vi "Periodic Tasks.vi"(8 "error in":errorcluster) -> ()   [LabVIEW 2011]
doc: "This VI runs in parallel to other tasks. It can contain as many user-defined periodic loops as you need. These can carry out PID or other sorts of timed response."
uses:
  <vilib>/Rock Robotics/SystemInterfaces/Typedef/FPGA_TypedefDigitalModule.ctl
  ADXL345 I2C Range.ctl
  <vilib>/Rock Robotics/SystemInterfaces/Utilities/FPGA_UtilitiesLED Source.ctl
  <vilib>/Rock Robotics/SystemInterfaces/Utilities/FPGA_UtilitiesLED State.ctl
  <vilib>/Rock Robotics/WPI/Relay/WPI_RelayValue.ctl
  Robot Global Data.vi
  <vilib>/Utility/file.llb/Read From Spreadsheet File (string).vi
  <vilib>/addons/control/pid/pid.llb/PID (DBL).vi
  <vilib>/Rock Robotics/WPI/RobotDrive/WPI_RobotDriveArcadeDrive_Standard(NoSaturation).vi
  <vilib>/addons/control/pid/pid.llb/PID Output Rate Limiter (DBL).vi
  ADXL345 I2C Axis.ctl
  <vilib>/addons/control/pid/NI_PID_pid.lvlib
  <vilib>/Utility/file.llb/Write To Spreadsheet File (DBL).vi
panel:
  in  "BB A Delay":dbl=0.15
  in  "Coll Loop TIme":u32=50
  in  "Save Data":bool
  in  "Tip Tol 2":dbl
  in  "K Deriv 2":dbl
  in  "K Prop 2":dbl
  in  "Reset Sonar 4":bool
  in  "Reset Sonar 3":bool
  in  "Motor C":dbl=-1.0
  in  "time":dbl
  in  "Dial":i64(knob)=50 scale=0.0..500.0
  in  "error":dbl(knob) scale=-0.5..0.5
  out "L Sonar":cluster{dbl, "Filtered":dbl}(graph)
  out "R Sonar":cluster{dbl, "Filtered":dbl}(graph)
  out "Gain (VoltsPerDegree/Second)":dbl
  out "Gain":dbl
  out "Left Enc":dbl
  out "Right Enc":dbl
  out "Right Wheel Encoder":dbl
  out "Left Wheel Encoder":dbl
  out "output 2":dbl format="%.2f"
  out "output":dbl format="%.2f"
  out "MAC Address":string
  out "Personality":string
  in  "Number Samples to Average":u8(knob)=30 min=1 max=128 scale=0.0..30.0
  in  "Minimum Rate":dbl(knob)=10.067348623787787 scale=0.0..20.0
  out "Angle":dbl
  in  "Tab Control":T1(tab)
  out "Z axis":dbl(slide) scale=-1.0..1.0
  out "Y AXIS":dbl(slide) scale=-1.0..1.0
  out "X AXIS":dbl(slide) scale=-1.0..1.0
  out "R Mode":bool
  out "L Mode":bool
  in  "Sonar Offset":dbl(knob)=-0.020166607778801193 scale=-20.0..20.0
  in  "Sonar Scale":dbl(knob)=102.7182978218157 scale=80.0..120.0
  in  "Rate Thresh":dbl(knob)=100.27914654140737 step=0.001 scale=0.0..200.0
  out "Right Sonar":dbl
  out "Left Sonar":dbl
  out "R Filtered":dbl
  out "L Filtered":dbl
  out "R OOR":bool
  out "L OOR":bool
  out "hi limit":dbl=70.0
  in  "Hyster":dbl=0.3 step=0.1
  out "Valid Target":bool
  out "Stable":bool
  out "Intake":bool
  out "Steering":bool
  in  "Close":dbl=13.0
  out "Close?":bool
  in  "DS time":dbl=2.0
  in  "x":dbl=12.0
  in  "Balance 2":dbl=0.07
  in  "Gain 2":dbl=0.6 step=0.05
  in  "Base":dbl=0.8 step=0.1
  out "Left Motor Sonar":dbl=36.0
  out "Right Motor Sonar":dbl=36.0
  in  "IR Delay (sec)":dbl(knob)=0.20745032848680972 scale=0.0..1.0
  in  "Intake Delay (sec)":dbl(knob)=0.15160369527651382 scale=0.0..1.0
  out "error":dbl
  out "dist":dbl
  out "Sonar State":i32
  in  "Reset Sonar":bool
  out "Kick State":i32
  in  "Sonar Loop":bool
  in  "ms multiple":u32=50
  in  "DIO Module":T2
  in  "Range":T3 items=["+/- 2 g", "+/- 4 g", "+/- 8 g", "+/- 16 g"]
  out "Z Axis Accel":dbl
  out "Y Axis Accel":dbl
  out "X Axis Accel":dbl
  in  "stop":bool
  out "Loop":i32
  out "X Axis":dbl(knob) scale=-2.0..2.0
  out "Y Axis":dbl(knob) scale=-2.0..2.0
  out "Z Axis":dbl(knob) scale=-2.0..2.0
  out "Up ?":bool
  out "K Prop":dbl=0.04035443158900818
  out "Balance":cluster{"setpoint":dbl, "GYRO":dbl}(graph)
  in  "Bal Tol":dbl=2.0
  in  "Coerce":dbl=0.5
  out "Drive":dbl
  out "In Tol?":bool
  out "Tip Tol":dbl=2.25 step=0.01
  in  "Motor Add":dbl=0.1
  out "Pitch Angle":dbl
  out "Gain (VoltsPerDegree/Second) 2":dbl
  in  "reset":bool=TRUE
  in  "DRIFT (Deg/sec)":dbl(knob) scale=-0.3..0.3
  out "K Deriv":dbl=0.001046187815623034
  out "K Prop 2":dbl
  out "K Deriv 2":dbl
  out "Motor Add":dbl
  out "Coerce":dbl
  out "Bal Tol":dbl
  out "Tip Tol 2":dbl
  in  "T Ang Mult":dbl=-44.91
  in  "Turret Home Position":dbl=-180.0
  out "Turret Home Adjust":dbl
  out "Turret Yaw":dbl
  out "Turret Home":bool
  out "Read Right Limit":dbl=30.0
  out "Read Left Limit":dbl=-185.0
  in  "Motor Cuttout":dbl=0.06
  out "Motor is Cut Out":bool
  out "Turret Enc":dbl
  in  "Set Left Comp":dbl=-190.0
  in  "Set Right Comp":dbl=30.0
  in  "Speed near Limit":dbl=0.2
  in  "Near Limit (deg)":dbl=10.0
  out "Motor Command":dbl=0.04
  out "Softstop Override":bool
  in  "Set Left Test":dbl=-205.0
  in  "Set Right Test":dbl=30.0
  out "Left Limit":bool
  out "Right Limit":bool
  out "PB":bool
  out "Left Output":dbl format="%.2f"
  out "Left PID Out":dbl(graph)
  out "Left Brake Control Response":cluster{"setpoint":dbl, "Angle":dbl}(graph)
  in  "Deriv 2":dbl(knob)=0.0006002534638116536 scale=0.0..0.01
  in  "Int 2":dbl(knob) scale=0.0..0.2
  in  "Prop 2":dbl(knob)=0.18717165980295236 scale=0.0..0.5
  out "Right Output":dbl format="%.2f"
  in  "Brake Motor Add":dbl=0.05
  in  "Brake Motor Deadband":dbl=0.1
  in  "Brake Bump":i64=1
  in  "Bump rate":dbl=400.0 format="%.2f"
  in  "Shooter Loop milliseconds":u32=20
  in  "Shooter Stable Tol (sec)":dbl(knob)=0.5029660632222493 scale=0.0..1.0
  out "Motor Command":dbl(slide) scale=0.0..1.0
  out "RPM In Tol ?":bool
  out "RPM Stable ?":bool
  out "Distance":dbl
  out "Frame":i32
  out "Angle 2":dbl
  out "Valid Target 2":bool
  in  "Momen Time (sec)":dbl(knob) scale=0.0..0.1
  out "Bridge Down":bool
  out "Bridge Up":bool
  in  "Servo Unlock":i16=34
  in  "Wait for Servo (ms)":u32=500
  out "Mode":i32
  in  "Deriv":dbl(knob)=0.030506642412339725 scale=0.0..0.01
  in  "Int":dbl(knob) scale=0.0..0.2
  in  "Prop":dbl(knob)=0.059181315414781936 scale=0.0..0.5
  out "Bot Turn Control Response":cluster{"setpoint":dbl, "Angle":dbl}(graph)
  out "PID Output":dbl(graph)
  in  "Turn Rate":dbl(knob)=0.07001503420246988 scale=0.0..1.0
  in  "Turn To":dbl(knob)=0.07001503420246988 scale=-360.0..360.0
  out "Output":dbl format="%.2f"
  out "Turn":bool
  out "Robot Gyro":dbl
  in  "Test Turret DB":dbl(knob) scale=-0.2..0.2
  out "Turret Ready?":bool
  in  "Turret Stable Tol (sec)":dbl(knob)=0.7049412817911537 scale=0.0..4.0
  out "Turret Stable?":bool
  out "Motor Output":dbl(knob) scale=-0.5..0.5
  in  "Test?":bool
  in  "Intake Speed":dbl(knob)=1.0 scale=-1.0..1.0
  in  "Fire Conv Speed":dbl(knob)=0.49108018984762314 scale=-1.0..1.0
  in  "Prime Conv Speed":dbl(knob)=0.20488113025200594 scale=-1.0..1.0
  out "Compressor Running":bool
  out "error out":errorcluster
  out "error out 2":errorcluster
  out "error out 3":errorcluster
  # "Compass"
  # "Gyro"
  # "If bridge crashes down after Tip, reduce Tip Tol\nuntil high end does not strike floor.\nThen, if bot backs up too far, increase K Deriv and \nmaybe increase Bal Tol.  This assumes a gyro 0 ref not drifting."
  # "File Read:"
  # "Set To:"
  # "Ches T Angle Multiplier = -44.91"
  # "LL is -190"
  # "RL is +30"
  # "Competition Bot Values"
  # "Fairgrounds Test Bot was 0.35 sec\nCheas Start was 0.5 sec"
  # "P: 0.06, I: 0.0, D: 0.03"
  # "To adjust Turret Motor deadband limits, use test button and dial.  Set values in Turret VI front panel.\nMotor Cuttout in this Turret Encoding Tab should be set to 0.0 during this testing."
  # "CW"
  # "CCW"
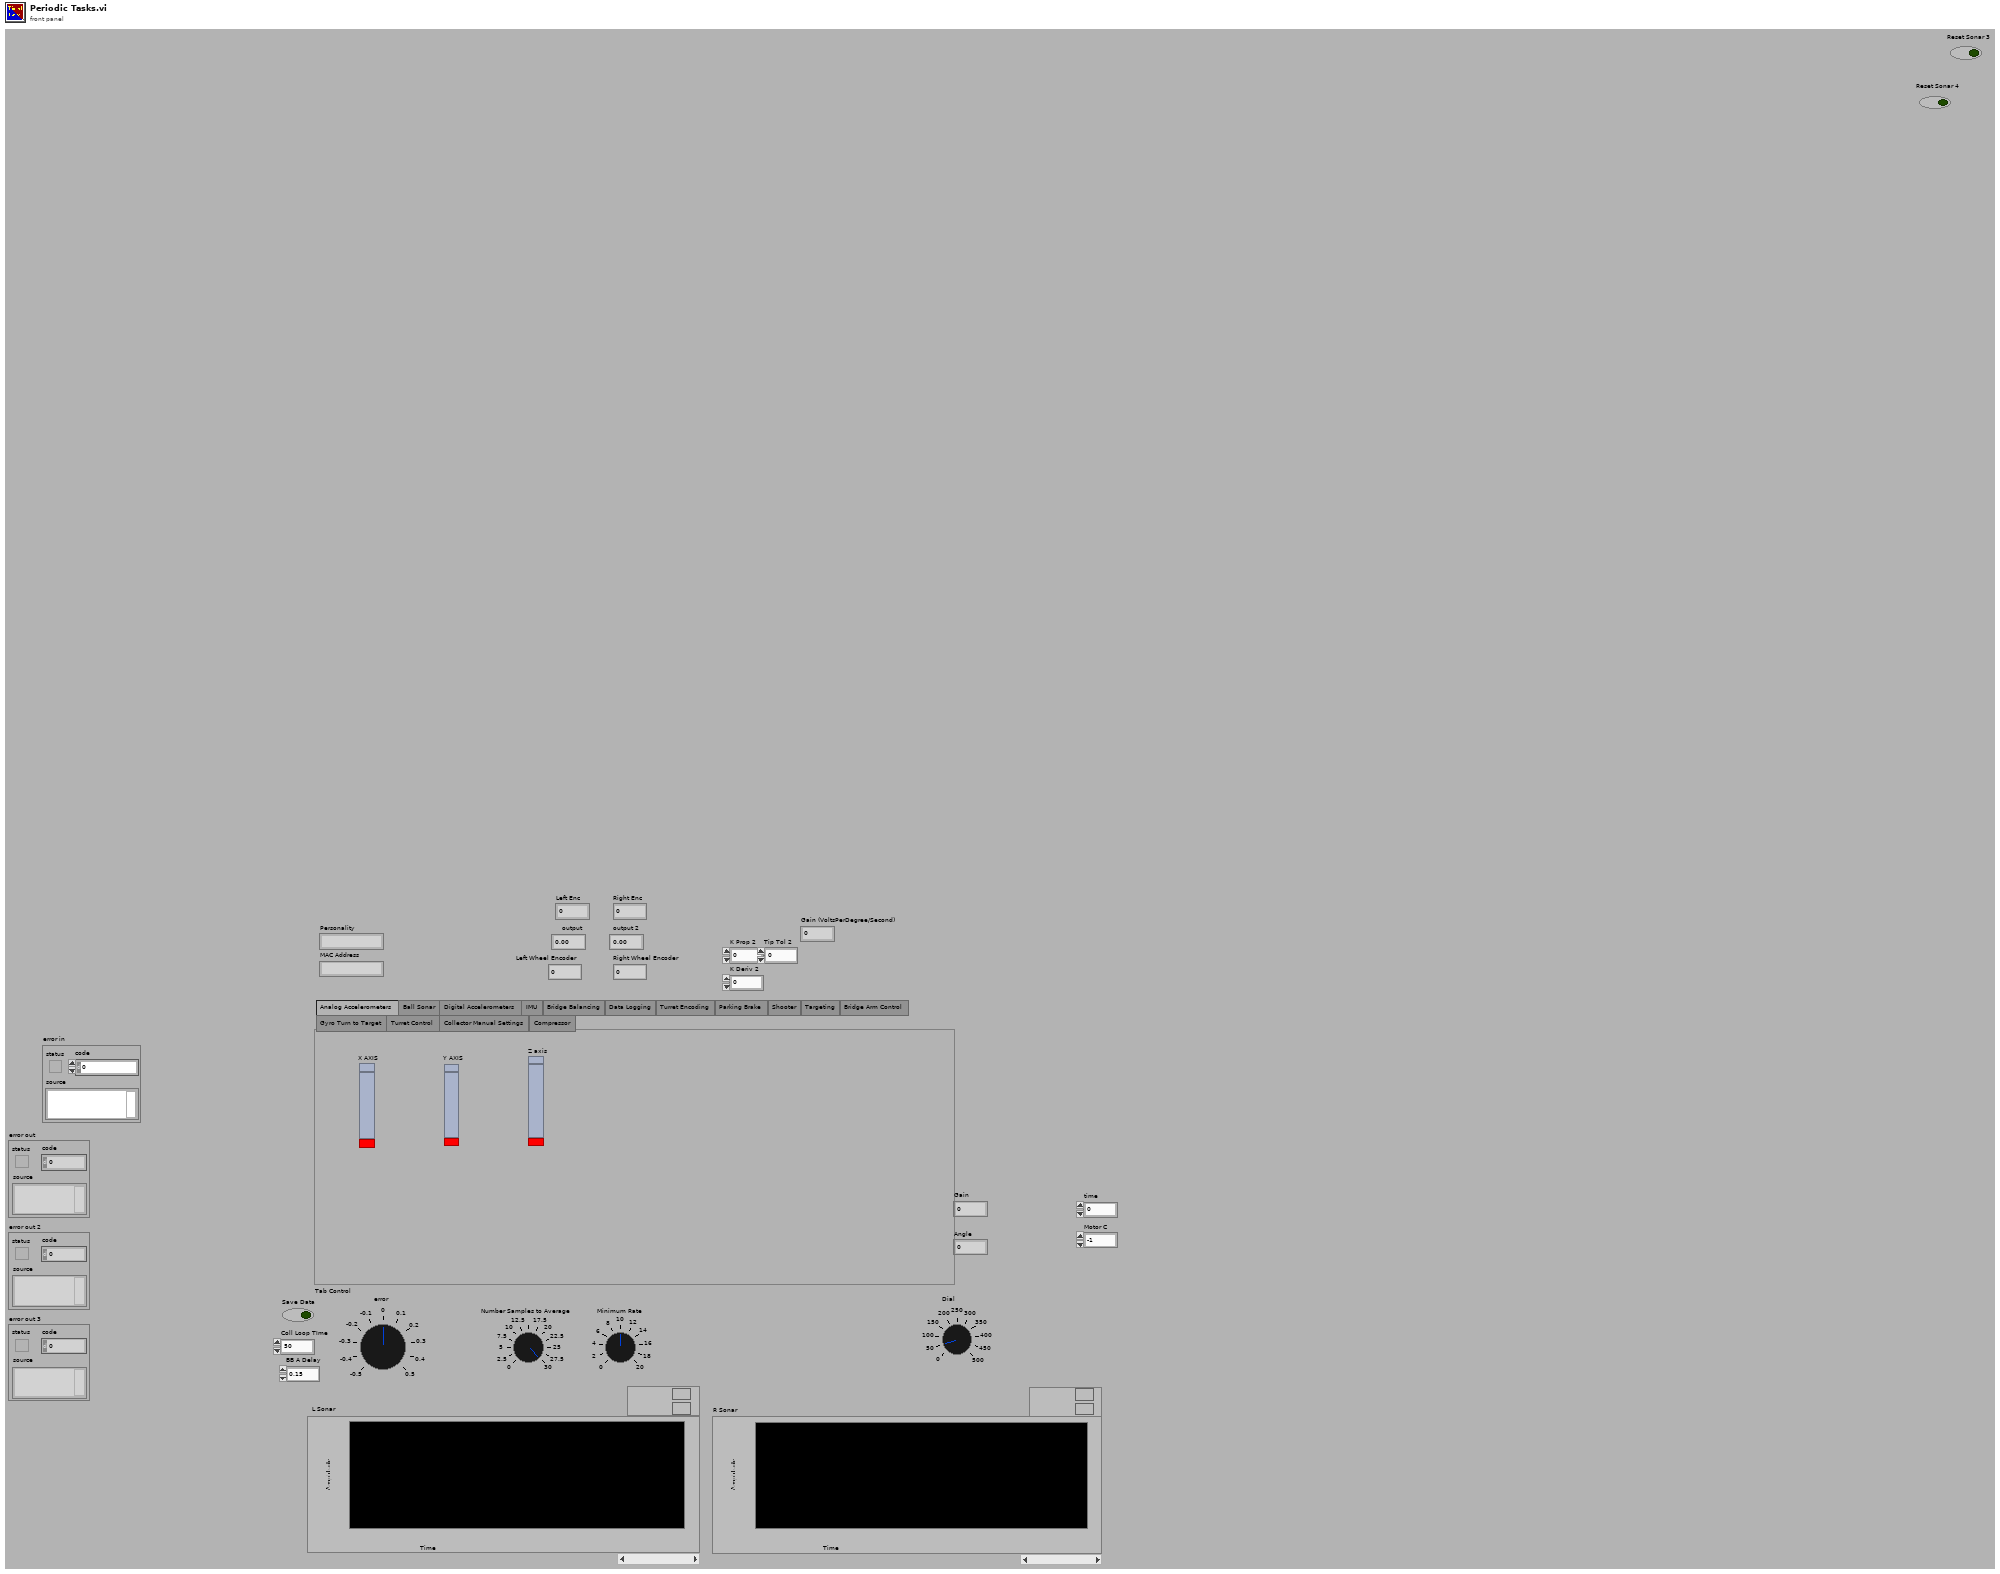
[diagram p1: front panel]
types:
  T1 = enum32{"Analog Accelerometers", "Ball Sonar", "Digital Accelerometers", "IMU", "Bridge Balancing", "Data Logging", "Turret Encoding", "Parking Brake", "Shooter", "Targeting", "Bridge Arm Control", "Gyro Turn to Target", "Turret Control", "Collector Manual Settings", "Compressor"}
  T2 = typedef "FPGA_TypedefDigitalModule.ctl" = enum16{"Digital Module 1", "Digital Module 2"}
  T3 = typedef "ADXL345 I2C Range.ctl" = u8
  T4 = typedef "WPI_ServoDeviceRef.ctl" = cluster{"DeviceStatus":errorcluster, "Digital Module":T2, "PWM Channel":T5, "DeadBand":T6}
  T5 = typedef "FPGA_DIOPWMChannel.ctl" = enum8{"PWM 1", "PWM 2", "PWM 3", "PWM 4", "PWM 5", "PWM 6", "PWM 7", "PWM 8", "PWM 9", "PWM 10", "Invalid"}
  T6 = typedef "WPI_PWMDeadband.ctl" = cluster{"Name":string, "maxPositivePwm":i32, "minPositivePwm":i32, "centerPwm":i32, "maxNegativePwm":i32, "minNegativePwm":i32, "angularRange":u16}
  T7 = typedef "WPI_DigitalInputDevRef.ctl" = cluster{"DevStatus":errorcluster, "DIO Channel":T8, "Digital Module":T2}
  T8 = typedef "FPGA_DIOChannel.ctl" = enum8{"DIO 1", "DIO 2", "DIO 3", "DIO 4", "DIO 5", "DIO 6", "DIO 7", "DIO 8", "DIO 9", "DIO 10", "DIO 11", "DIO 12", "DIO 13", "DIO 14", "Invalid"}
  T9 = typedef "WPI_RelayDevRef.ctl" = cluster{"DevStatus":errorcluster, "Relay Channel":T10, "Digital Module":T2, "Relay Direction":T11}
  T10 = typedef "FPGA_DIORelayChannel.ctl" = enum8{"Relay 1", "Relay 2", "Relay 3", "Relay 4", "Relay 5", "Relay 6", "Relay 7", "Relay 8", "Invalid"}
  T11 = typedef "WPI_RelayDirection.ctl" = enum16{"Both directions", "Forward only", "Reverse only"}
  T12 = typedef "WPI_RelayValue.ctl" = enum16{"Off", "On", "Forward", "Reverse"}
  T13 = typedef "WPI_EncoderDevRef.ctl" = cluster{"DevStatus":errorcluster, "EncoderIndex":T14, "CounterIndex":T15, "DistancePerCount":dbl, "Decoding Type":T16}
  T14 = typedef "FPGA_EncoderIdx.ctl" = enum8{"Enc 0", "Enc 1", "Enc 2", "Enc 3", "Invalid"}
  T15 = typedef "FPGA_CounterCtrSystemIndex.ctl" = enum8{"Ctr 0", "Ctr 1", "Ctr 2", "Ctr 3", "Ctr 4", "Ctr 5", "Ctr 6", "Ctr 7", "Invalid"}
  T16 = typedef "WPI_EncoderType.ctl" = enum16{"1x", "2x", "4x"}
  T17 = typedef "WPI_AccelerometerDevRef.ctl" = cluster{"DevStatus":errorcluster, "Analog Module":T18, "Analog Channel":T19, "Scaling":T20}
  T18 = typedef "FPGA_TypedefAnalogModule.ctl" = enum16{"Analog Module 1", "Analog Module 2"}
  T19 = typedef "FPGA_AIChannel.ctl" = enum8{"AI 1", "AI 2", "AI 3", "AI 4", "AI 5", "AI 6", "AI 7", "AI 8", "Invalid"}
  T20 = typedef "WPI_AccelerometerScaling.ctl" = cluster{"Gain (VoltsPerG)":dbl, "Center Voltage":dbl}
  T21 = typedef "FPGA_UtilitiesLED State.ctl" = enum16{"Off", "On", "Toggle"}
  T22 = typedef "FPGA_UtilitiesLED Source.ctl" = enum16{"User LED", "FPGA LED"}
  T23 = typedef "WPI_CompressorDevRef.ctl" = cluster{"DevStatus":errorcluster, "DigitalInputDevRef":T7, "RelayDevRef":T9}
  T24 = typedef "WPI_GyroDevRef.ctl" = cluster{"DevStatus":errorcluster, "Analog Module":T18, "Analog Channel":T19, "Offset":dbl, "Gain (VoltsPerDegree/Second)":dbl}
  T25 = typedef "WPI_I2CDevRef.ctl" = cluster{"DevStatus":errorcluster, "Digital Module":T2, "Device Address":u8}
  T26 = typedef "ADXL345 I2C Axis.ctl" = u8
  T27 = typedef "WPI_CounterDevRef.ctl" = cluster{"DevStatus":errorcluster, "CntIndex":T15}
  T28 = enum16{"open", "replace", "create", "open or create", "replace or create", "replace or create with confirmation"}
  T29 = typedef "WPI_MotorControlDeviceRef.ctl" = cluster{"DeviceStatus":errorcluster, "Type":enum16{"PWM", "CAN"}, "PWM":cluster{"Digital Module":T2, "PWM Channel":T5, "DeadBand":T6}, "CAN":cluster{"Device Number":u8, "Control Mode":T30, "Semaphore":T31, "Max Vout":dbl}, "Invert":bool, "TransformRef":T32, "InvTransformRef":T32}
  T30 = typedef "WPI_CANJaguar_ControlMode.ctl" = enum8{"Percent VBus", "Current", "Speed", "Position", "Voltage"}
  T31 = typedef "Semaphore RefNum" = refnum<k1>
  T32 = typedef "WPI_PWMTransform_ConPane.ctl" = refnum<vi>
  T33 = typedef "WPI_AnalogChannelDevRef.ctl" = cluster{"DevStatus":errorcluster, "Analog Module":T18, "Analog Channel":T19}
  T34 = cluster{dbl, dbl, dbl, "Filtered":dbl, "Filtered":dbl, dbl, dbl, dbl, dbl, dbl, dbl}
  T35 = cluster{"all rows[0]":string, "all rows[1]":string, "all rows[2]":string, "all rows[3]":string, "all rows[4]":string, "all rows[5]":string, "all rows[6]":string, "all rows[7]":string, "all rows[8]":string}
  T36 = cluster{"Frame":i32, "Distance":dbl, dbl, "Valid Target":bool}
  T37 = typedef "WPI_RobotDriveDevRef.ctl" = cluster{"DevStatus":errorcluster, "Motors[]":T29[], "Square Inputs":bool, "Max Output":dbl, "Isochronous":bool}
  T38 = cluster{"Left Wheel Encoder":dbl, "Left Wheel Encoder":dbl}
  T39 = cluster{"Prop 2":dbl, "Int 2":dbl, "Deriv 2":dbl}
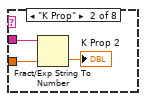
[diagram p3: hidden frame]
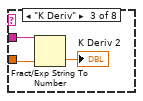
[diagram p4: hidden frame]
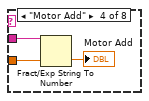
[diagram p5: hidden frame]
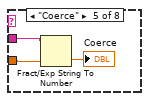
[diagram p6: hidden frame]
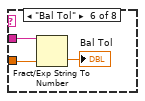
[diagram p7: hidden frame]
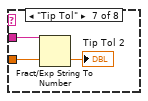
[diagram p8: hidden frame]
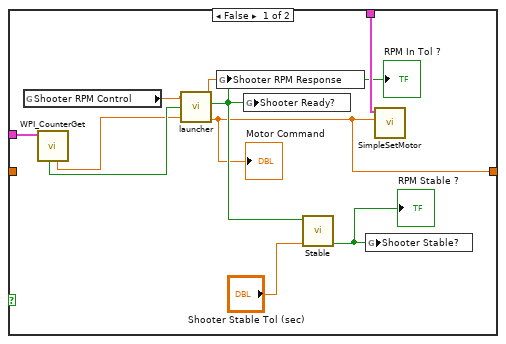
[diagram p9: hidden frame]
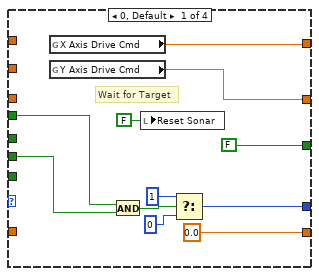
[diagram p15: hidden frame]
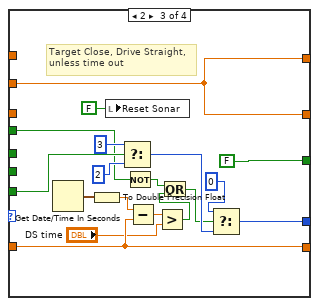
[diagram p16: hidden frame]
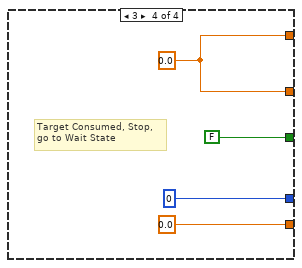
[diagram p17: hidden frame]
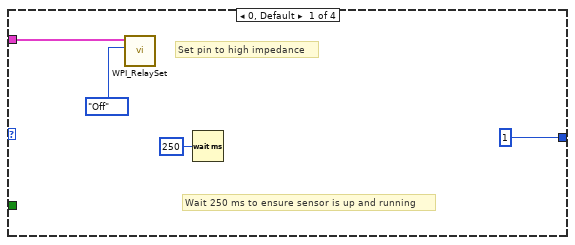
[diagram p19: hidden frame]
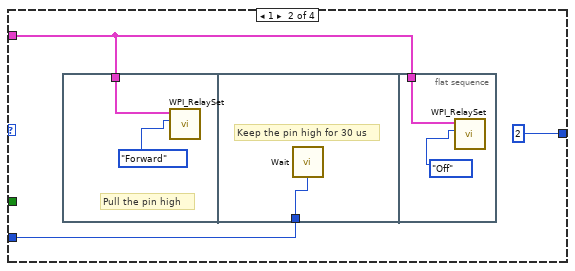
[diagram p20: hidden frame]
diagram:
  w57 = 0.0
  w59 = FALSE  # Valid Target
  w56 = 17.0  # Distance
  w58 = -1  # Frame
  w67 = u16 1130  # port
  (unwired) "If using the compressor, you should\nplace the control loop in parallel with\nthe existing loops, such as in this\ncommented code. Since the VI loops internally, you don't need to place it in an additional loop."
  (unwired) "This code flashes the USER1 LED on the cRIO.  It is a simple way to let you know your code is running on the cRIO.  You can leave this code if you find it helpful, or delete it if you don't want it."
  (unwired) "This VI is a good place to take care of periodic tasks such as control loops.\n\nAdd code to the existing loops, or duplicate a loop to define a new rate. You can allocate I/O references here, or in Begin.vi.\n\nPeriodic loops will often operate with setpoints from other loops. Use a global variable such as Robot Global Data for sharing data between loops."
  # "0 - Start\n1 - Kick\n2 - Run\n3 - Reset"
  # "Drive, Brake, Fetch, & Balance System"
  n1 = call <vilib>:"WPI_ServoRefNum Registry Get.vi"("refnum name"="Bridge Lock Servo") -> ("ServoDeviceRef"=w37:T4)  [unwired: 1 in, 9 out]
  n2 = First Call?() -> (First Call?: T/F=w38:bool)
  n3 = case shown="True" w38 {
    tunnel: w37 -> [_ w104]
    frame False {
    }
    frame True {
      n4 = call <vilib>:"WPI_ServoSetAngle.vi"("Angle"=0, "ServoDeviceRef"=w104) -> ()  [unwired: 1 in, 9 out]
    }
  }
  n5 = call <vilib>:"WPI_DigitalInputRefNum Registry Get.vi"("refnum name"="Bridge Actuator Up") -> ("DigitalInputDevRef"=w42:T7)  [unwired: 9 in, 1 out]
  n6 = call <vilib>:"WPI_DigitalInputRefNum Registry Get.vi"("refnum name"="Bridge Actuator Down") -> ("DigitalInputDevRef"=w43:T7)  [unwired: 9 in, 1 out]
  n7 = call <vilib>:"WPI_RelayRefNum Registry Get.vi"("refnum name"="Bridge Actuator") -> ("RelayDevRef"=w39:T9)  [unwired: 9 in, 1 out]
  n8 = while {
    tunnel: w43 -> [w123]
    tunnel: w42 -> [w122]
    tunnel: w37 -> [w120]
    tunnel: w39 -> [w121]
    stop <- FALSE stop-if-true
    # "Bridge Arm Up"
    # "Bridge Arm Down"
    n9 = call <vilib>:"WPI_DigitalInputGetValue.vi"("DigitalInputDevRef"=w122) -> ("Value"=w117:bool)  [unwired: 8 in, 2 out]
    n10 = call <vilib>:"WPI_DigitalInputGetValue.vi"("DigitalInputDevRef"=w123) -> ("Value"=w118:bool)  [unwired: 8 in, 2 out]
    n11 = Not(x=w117) -> (.not. x?=→"Bridge Up":bool)
    n12 = Not(x=w118) -> (.not. x?=→"Bridge Down":bool)
    n13 = global read "Robot Global Data.vi" "Dr Button 2"() -> (w119:bool)
    n14 = global read "Robot Global Data.vi" "Dr Button 1"() -> (w115:bool)
    n15 = And(x=w118, y=w119) -> (x .and. y?=w107:bool)
    n16 = And(x=w117, y=w115) -> (x .and. y?=w106:bool)
    n17 = feedback #1(FALSE) -> (w113:bool)
    n18 = Less?(x=w106, y=w113) -> (x < y?=w111:bool)
    n19 = feedback-in #1(w106) -> ()
    n20 = feedback #2(FALSE) -> (w109:bool)
    n21 = Less?(x=w107, y=w109) -> (x < y?=w108:bool)
    n22 = feedback-in #2(w107) -> ()
    n23 = case shown="False" w107 {
      tunnel: w106 -> [w127 _]
      tunnel: w120 -> [w128 _]
      tunnel: w121 -> [w129 w205]
      tunnel: w111 -> [w126 _]
      tunnel: w108 -> [w125 _]
      frame False {
        n24 = case shown="False" w127 {
          tunnel: w129 -> [w137 w178]
          tunnel: w128 -> [_ w185]
          tunnel: w126 -> [w135 _]
          tunnel: w125 -> [w134 _]
          frame False {
            # "Momentum Killer State Machine"
            # "0: Init\n1: Brake to stop up\n2: Stop\n3: Brake to stop dn"
            # "Up"
            # "Dn"
            # "Bridge Arm Stopped"
            # "No Request"
            n25 = feedback #3() -> (w131:dbl)  [unwired: 1 in]
            n26 = feedback #4(0 ("t")) -> (w130:i32)
            "Mode" <- w130
            n27 = case shown="0, Default" w130 {
              tunnel: w137 -> [w139 w158 w162 w165]
              tunnel: [w148 w157 0 ("t") w169] -> w136
              tunnel: w135 -> [w146 _ _ _]
              tunnel: w134 -> [w140 _ _ _]
              tunnel: [w144 w154 0.0 w168] -> w132
              tunnel: w131 -> [_ w154 _ w168]
              frame 0, Default {
                n28 = call <vilib>:"WPI_RelaySet.vi"("RelayValue"=WPI_RelayValue."Off", "RelayDevRef"=w139) -> ()  [unwired: 8 in, 2 out]
                n29 = Get Date/Time In Seconds() -> (seconds since 1Jan1904=w145:timestamp)
                n30 = Select(t=3, s=w140, f=0) -> (s? t:f=w141:i32)
                n31 = To Double Precision Float(number=w145) -> (double precision float=w144:dbl)
                n32 = Select(t=1, s=w146, f=w141) -> (s? t:f=w148:i32)
              }
              frame 1 {
                n33 = Get Date/Time In Seconds() -> (seconds since 1Jan1904=w153:timestamp)
                n34 = call <vilib>:"WPI_RelaySet.vi"("RelayValue"=WPI_RelayValue."Reverse", "RelayDevRef"=w158) -> ()  [unwired: 8 in, 2 out]
                n35 = To Double Precision Float(number=w153) -> (double precision float=w150:dbl)
                n36 = Add(x=w154, y="Momen Time (sec)") -> (x+y=w151:dbl)
                n37 = Greater Or Equal?(x=w150, y=w151) -> (x >= y?=w152:bool)
                n38 = Select(t=2, s=w152, f=1) -> (s? t:f=w157:i32)
              }
              frame 2 {
                n39 = call <vilib>:"WPI_RelaySet.vi"("RelayValue"=WPI_RelayValue."Off", "RelayDevRef"=w162) -> ()  [unwired: 8 in, 2 out]
              }
              frame 3 {
                # "Defeat Brake to stop Dn"
                n40 = Get Date/Time In Seconds() -> (seconds since 1Jan1904=w173:timestamp)
                n41 = call <vilib>:"WPI_RelaySet.vi"("RelayValue"=WPI_RelayValue."Off", "RelayDevRef"=w165) -> ()  [unwired: 8 in, 2 out]
                n42 = To Double Precision Float(number=w173) -> (double precision float=w166:dbl)
                n43 = Add(x=w168, y=0.0) -> (x+y=w167:dbl)
                n44 = Greater Or Equal?(x=w166, y=w167) -> (x >= y?=w174:bool)
                n45 = Select(t=2, s=w174, f=3) -> (s? t:f=w169:i32)
              }
            }
            n46 = feedback-in #3(w132) -> ()
            n47 = feedback-in #4(w136) -> ()
          }
          frame True {
            # "Requesting Up"
            n48 = flat-sequence {
              tunnel: [w190] -> w184
              tunnel: [w189] -> w183
              tunnel: [w188] -> w182
              tunnel: w185 -> [w187]
              tunnel: [w196] -> w181
              tunnel: w184 -> [w196]
              tunnel: [w195] -> w180
              tunnel: w183 -> [w195]
              tunnel: w182 -> [w194]
              tunnel: [w194] -> w179
              tunnel: w181 -> [w199]
              tunnel: w180 -> [w198]
              tunnel: w179 -> [w197]
              tunnel: w178 -> [w200]
              tunnel: [w199] -> w177
              tunnel: [w198] -> w176
              tunnel: [w197] -> w175
              tunnel: w177 -> [w204]
              tunnel: w176 -> [w203]
              tunnel: w175 -> [w202]
              frame #0 {
                n49 = call <vilib>:"WPI_ServoGetAngle.vi"("ServoDeviceRef"=w187) -> ("ServoDeviceRef"=w191:T4, "Angle"=w188:u16, "error out"=w192:errorcluster)  [unwired: 1 in, 6 out]
                n50 = call <vilib>:"WPI_ServoSetAngle.vi"("error in (no error)"=w192, "Angle"="Servo Unlock", "ServoDeviceRef"=w191) -> ("error out"=w189:errorcluster, "ServoDeviceRef"=w190:T4)  [unwired: 7 out]
              }
              frame #1 {
                n51 = Wait (ms)(milliseconds to wait="Wait for Servo (ms)") -> ()  [unwired: 1 out]
              }
              frame #2 {
                n52 = call <vilib>:"WPI_RelaySet.vi"("RelayValue"=WPI_RelayValue."Forward", "RelayDevRef"=w200) -> ()  [unwired: 8 in, 2 out]
              }
              frame #3 {
                n53 = call <vilib>:"WPI_ServoSetAngle.vi"("error in (no error)"=w203, "Angle"=w202, "ServoDeviceRef"=w204) -> ()  [unwired: 9 out]
              }
            }
          }
        }
      }
      frame True {
        # "Requesting Down"
        n54 = call <vilib>:"WPI_RelaySet.vi"("RelayValue"=WPI_RelayValue."Reverse", "RelayDevRef"=w205) -> ()  [unwired: 8 in, 2 out]
      }
    }
    n55 = Wait (ms)(milliseconds to wait=u32 40) -> ()  [unwired: 1 out]
  }
  n56 = local write "Read Right Limit"(inf) -> ()
  n57 = local write "Read Left Limit"(-inf) -> ()
  n58 = call <vilib>:"WPI_DigitalInputRefNum Registry Get.vi"("refnum name"="Turret Home") -> ("DigitalInputDevRef"=w94:T7)  [unwired: 9 in, 1 out]
  n59 = call <vilib>:"WPI_EncoderRefNum Registry Get.vi"("refnum name"="Left Wheel Encoder") -> ("EncoderDevRef"=w100:T13)  [unwired: 9 in, 1 out]
  n60 = call <vilib>:"WPI_EncoderRefNum Registry Get.vi"("refnum name"="Right Wheel Encoder") -> ("EncoderDevRef"=w99:T13)  [unwired: 9 in, 1 out]
  n61 = disable-structure shown="Disabled" {
    frame Disabled {
      n62 = call <vilib>:"WPI_AccelerometerRefNum Registry Get.vi"("refnum name"="x Accel") -> ("AccelerometerDevRef"=w210:T17)  [unwired: 9 in, 1 out]
      n63 = call <vilib>:"WPI_AccelerometerRefNum Registry Get.vi"("refnum name"="Y Accel") -> ("AccelerometerDevRef"=w209:T17)  [unwired: 9 in, 1 out]
      n64 = call <vilib>:"WPI_AccelerometerRefNum Registry Get.vi"("refnum name"="Z Accel") -> ("AccelerometerDevRef"=w207:T17)  [unwired: 9 in, 1 out]
      n65 = while {
        tunnel: w210 -> [w216]
        tunnel: w209 -> [w215]
        tunnel: w207 -> [w213]
        stop <- FALSE stop-if-true
        n66 = call <vilib>:"WPI_AccelerometerGetAcceleration.vi"("AccelerometerDevRef"=w215) -> ("Acceleration"=→"Y AXIS":dbl)  [unwired: 8 in, 2 out]
        n67 = call <vilib>:"WPI_AccelerometerGetAcceleration.vi"("AccelerometerDevRef"=w213) -> ("Acceleration"=→"Z axis":dbl)  [unwired: 8 in, 2 out]
        n68 = call <vilib>:"WPI_AccelerometerGetAcceleration.vi"("AccelerometerDevRef"=w216) -> ("Acceleration"=→"X AXIS":dbl)  [unwired: 8 in, 2 out]
        n69 = Wait (ms)(milliseconds to wait=u32 10) -> ()  [unwired: 1 out]
      }
    }
    frame Enabled {
    }
  }
  n70 = while {
    tunnel: w100 -> [w229]
    tunnel: w99 -> [w228]
    tunnel: "Turret Encoder" ("refnum name") -> [w239]
    tunnel: w94 -> [w238]
    stop <- FALSE stop-if-true
    n71 = global read "Robot Global Data.vi" "Personality"() -> (w223:string)
    n72 = call <vilib>:"WPI_EncoderConfigureTimer.vi"("Number Samples to Average"="Number Samples to Average", "Minimum Rate"="Minimum Rate", "EncoderDevRef"=w229) -> ("EncoderDevRef"=w231:T13)  [unwired: 1 in, 7 out]
    n73 = call <vilib>:"WPI_EncoderConfigureTimer.vi"("Number Samples to Average"="Number Samples to Average", "Minimum Rate"="Minimum Rate", "EncoderDevRef"=w228) -> ("EncoderDevRef"=w230:T13)  [unwired: 1 in, 7 out]
    n74 = Equal?(x=w223, y="Sting") -> (x = y?=w221:bool)
    n75 = call <vilib>:"WPI_EncoderGet.vi"("EncoderDevRef"=w231) -> ("Distance"=w247:dbl)  [unwired: 5 in, 5 out]
    n76 = call <vilib>:"WPI_EncoderGet.vi"("EncoderDevRef"=w230) -> ("Distance"=w246:dbl)  [unwired: 5 in, 5 out]
    n77 = call <vilib>:"WPI_DigitalInputGetValue.vi"("DigitalInputDevRef"=w238) -> ("Value"=w233:bool)  [unwired: 8 in, 2 out]
    "Turret Home" <- w233
    n78 = case shown="True" w221 {
      tunnel: ["Set Left Test" "Set Left Comp"] -> w225
      tunnel: ["Set Right Test" "Set Right Comp"] -> w224
      frame False {
        # "Sister-Sting"
      }
      frame True {
        # "Sting"
      }
    }
    n79 = call "836Elevator_Encoder.vi"("Elevator Encoder Ref"=w239) -> ("Output"=w240:dbl)  [unwired: 1 in]
    "Turret Enc" <- w240
    n80 = global write "Robot Global Data.vi" "Turret Home"(w233) -> ()
    n81 = Multiply(x="T Ang Mult", y=w240) -> (x*y=w232:dbl)
    n82 = global write "Robot Global Data.vi" "Turret Encoder"(w240) -> ()
    n83 = Add(x=w247, y=w246) -> (x+y=w245:dbl)
    n84 = global write "Robot Global Data.vi" "Right Wheel Encoder"(w246) -> ()
    n85 = global write "Robot Global Data.vi" "Left Wheel Encoder"(w247) -> ()
    n86 = Divide(x=w245, y=2.0) -> (x/y=w243:dbl)
    n87 = feedback #5(0.0) -> (w236:dbl)
    n88 = case shown="True" w233 {
      tunnel: w232 -> [_ w257]
      tunnel: [w253 w256] -> w234
      tunnel: w236 -> [w253 _]
      tunnel: w225 -> [_ w255]
      tunnel: w224 -> [_ w254]
      frame False {
      }
      frame True {
        n89 = local write "Read Left Limit"(w255) -> ()
        n90 = local write "Read Right Limit"(w254) -> ()
        n91 = Subtract(x="Turret Home Position", y=w257) -> (x-y=w256:dbl)
        "Turret Home Adjust" <- w256
      }
    }
    n92 = Add(x=w232, y=w234) -> (x+y=w237:dbl)
    "Turret Yaw" <- w237
    n93 = feedback-in #5(w234) -> ()
    n94 = global write "Robot Global Data.vi" "Avg Wheel Encoder"(w243) -> ()
    n95 = global write "Robot Global Data.vi" "Turret Yaw"(w237) -> ()
    n96 = Wait Until Next ms Multiple(millisecond multiple=u32 10 ("milliseconds to wait")) -> ()  [unwired: 1 out]
  }
  n97 = while {
    stop <- FALSE stop-if-true
    # "This global is written to in the Autonomous and Teleop VIs"
    # "Flash the USER1 LED with the rate controlled from Autonomous and Teleop"
    n98 = global read "Robot Global Data.vi" "LED toggle rate (ms)"() -> (w259:u32)
    n99 = call <vilib>:"WPI_UtilitiesFRC LEDs.vi"("State"=FPGA_UtilitiesLED_State."Toggle", "LED Type"=FPGA_UtilitiesLED_Source."User LED") -> ()  [unwired: 1 in, 9 out]
    n100 = Wait (ms)(milliseconds to wait=w259) -> ()  [unwired: 1 out]
  }
  n101 = disable-structure shown="Disabled" {
    frame Disabled {
      n102 = call <vilib>:"WPI_CompressorRefNum Registry Get.vi"("refnum name"="The name") -> ("CompressorDevRef"=w264:T23)  [unwired: 9 in, 1 out]
      n103 = call <vilib>:"WPI_CompressorControlLoop.vi"("CompressorDevRef"=w264) -> ()  [unwired: 11 in]
    }
    frame Enabled {
    }
  }
  n104 = while {
    tunnel: [w277] -> w28
    tunnel: [w269] -> w11
    tunnel: [w266] -> w8
    stop <- w275 stop-if-true
    # "Max Sonar Range"
    # "Test-Bot"
    # "Competition - Bot"
    # "Test-Bot"
    # "Competition - Bot"
    # "Robot Gyro Gain"
    # "Pitch Gyro Gain"
    # "Bot-B is 0.00555"
    # "Competion Bot is 0.00608"
    n105 = global read "Robot Global Data.vi" "Personality"() -> (w273:string)
    n106 = Equal?(x=w273, y="Sting") -> (x = y?=w267:bool)
    n107 = Select(t=-0.0072, s=w267, f=-0.0066) -> (s? t:f=w269:dbl)
    n108 = Select(t=0.00608 ("Gain (VoltsPerDegree/Second)"), s=w267, f=0.00555 ("Gain (VoltsPerDegree/Second)")) -> (s? t:f=w277:dbl)
    "Gain" <- w277
    n109 = Select(t=70.0, s=w267, f=80.0) -> (s? t:f=w266:dbl)
    n110 = Wait Until Next ms Multiple(millisecond multiple=u32 10 ("milliseconds to wait")) -> ()  [unwired: 1 out]
    n111 = Not Equal?(x=w273, y="") -> (x != y?=w275:bool)
  }
  n112 = call <vilib>:"WPI_GyroRefNum Registry Get.vi"("refnum name"="Robot Gyro") -> ("error out"=w50:errorcluster, "GyroDevRef"=w49:T24)  [unwired: 9 in]
  n113 = call <vilib>:"WPI_GyroRefNum Registry Get.vi"("refnum name"="Pitch Gyro") -> ("error out"=w15:errorcluster, "GyroDevRef"=w16:T24)  [unwired: 9 in]
  n114 = Get Date/Time In Seconds() -> (seconds since 1Jan1904=w10:timestamp)
  n115 = call <vilib>:"WPI_GyroReset.vi"("error in (no error)"=w50, "GyroDevRef"=w49) -> ("error out"=w47:errorcluster, "GyroDevRef"=w48:T24)  [unwired: 8 in]
  n116 = call <vilib>:"WPI_GyroReset.vi"("error in (no error)"=w15, "GyroDevRef"=w16) -> ("error out"=w12:errorcluster, "GyroDevRef"=w13:T24)  [unwired: 8 in]
  n117 = To Double Precision Float(number=w10) -> (double precision float=w9:dbl)
  n118 = disable-structure shown="Disabled" {
    frame Disabled {
      n119 = call "ADXL345 I2C Open.vi"("Range"="Range", "DIO Module (Slot 4)"="DIO Module") -> ("I2CDevRef"=w280:T25)  [unwired: 2 in, 7 out]
      n120 = while {
        shift-right: [w301] -> w288
        shift-left: w280 -> [w303]
        tunnel: [w292] -> w283
        tunnel: [w291] -> w281
        tunnel: w280 -> [w290]
        tunnel: w280 -> [w289]
        i -> [w297]
        stop <- w299 stop-if-true
        w293 = T26 2 items=["X-Axis", "Y-Axis", "Z-Axis"] ("Axis")
        w302 = T26 0 items=["X-Axis", "Y-Axis", "Z-Axis"] ("Axis")
        w295 = T26 1 items=["X-Axis", "Y-Axis", "Z-Axis"] ("Axis")
        # "small loop delay"
        n121 = call "ADXL345 I2C Read.vi"("Axis"=w295, "I2CDevRef"=w290) -> ("Acceleration"=→"Y Axis Accel" →"Y Axis":dbl, "I2CDevRef Out"=w292:T25)  [unwired: 1 in, 7 out]
        n122 = call "ADXL345 I2C Read.vi"("Axis"=w293, "I2CDevRef"=w289) -> ("Acceleration"=→"Z Axis Accel" →"Z Axis":dbl, "I2CDevRef Out"=w291:T25)  [unwired: 1 in, 7 out]
        n123 = call "ADXL345 I2C Read.vi"("Axis"=w302, "I2CDevRef"=w303) -> ("error out"=w300:errorcluster, "Acceleration"=→"X Axis Accel" →"X Axis":dbl, "I2CDevRef Out"=w301:T25)  [unwired: 1 in, 6 out]
        n124 = Unbundle By Name(w300) -> ("status"=w306:bool)
        n125 = Or(x=w306, y="stop") -> (x .or. y?=w299:bool)
        n126 = Wait (ms)(milliseconds to wait=u32 100) -> ()  [unwired: 1 out]
        "Loop" <- w297
      }
      n127 = call <vilib>:"WPI_I2CClose.vi"("I2CDevRef"=w288) -> ("error out"=→"error out":errorcluster)  [unwired: 1 in, 9 out]
      n128 = call <vilib>:"WPI_I2CClose.vi"("I2CDevRef"=w283) -> ("error out"=→"error out 2":errorcluster)  [unwired: 1 in, 9 out]
      n129 = call <vilib>:"WPI_I2CClose.vi"("I2CDevRef"=w281) -> ("error out"=→"error out 3":errorcluster)  [unwired: 1 in, 9 out]
    }
    frame Enabled {
    }
  }
  n130 = while {
    tunnel: w48 -> [w332]
    tunnel: w47 -> [w330]
    tunnel: w28 -> [w325]
    tunnel: w13 -> [w322]
    tunnel: w12 -> [w321]
    tunnel: w11 -> [w318]
    tunnel: w9 -> [w309]
    stop <- FALSE stop-if-true
    n131 = Get Date/Time In Seconds() -> (seconds since 1Jan1904=w317:timestamp)
    n132 = feedback #6(w309) -> (w310:dbl)
    n133 = To Double Precision Float(number=w317) -> (double precision float=w308:dbl)
    n134 = Select(t=w308, s="reset", f=w310) -> (s? t:f=w311:dbl)
    n135 = feedback-in #6(w311) -> ()
    n136 = Subtract(x=w308, y=w311) -> (x-y=w316:dbl)
    n137 = call <vilib>:"WPI_GyroSetGain.vi"("error in (no error)"=w330, "Gain (VoltsPerDegree/Second)"=w325, "GyroDevRef"=w332) -> ("error out"=w329:errorcluster, "GyroDevRef"=w331:T24)  [unwired: 7 in]
    n138 = call <vilib>:"WPI_GyroSetGain.vi"("error in (no error)"=w321, "Gain (VoltsPerDegree/Second)"=w318, "GyroDevRef"=w322) -> ("error out"=w319:errorcluster, "GyroDevRef"=w320:T24)  [unwired: 7 in]
    n139 = Multiply(x=w316, y="DRIFT (Deg/sec)") -> (x*y=w313:dbl)
    n140 = call <vilib>:"WPI_GyroGetAngle.vi"("error in (no error)"=w329, "GyroDevRef"=w331) -> ("Angle"=w328:dbl)  [unwired: 6 in, 3 out]
    "Angle" <- w328
    n141 = call <vilib>:"WPI_GyroGetAngle.vi"("error in (no error)"=w319, "GyroDevRef"=w320) -> ("Angle"=w314:dbl)  [unwired: 6 in, 3 out]
    n142 = Add(x=w314, y=w313) -> (x+y=w312:dbl)
    n143 = call "Gyro Angle.vi"("Mod"=360.0, "Input"=w328) -> ("Output"=w326:dbl)  [unwired: 9 in]
    n144 = call "Gyro Angle.vi"("Mod"=180.0, "Input"=w312) -> ("Output"=w323:dbl)  [unwired: 9 in]
    "Pitch Angle" <- w323
    n145 = global write "Robot Global Data.vi" "Robot Gyro"(w326) -> ()
    n146 = global write "Robot Global Data.vi" "Pitch Gyro"(w323) -> ()
    n147 = Wait Until Next ms Multiple(millisecond multiple=u32 10 ("milliseconds to wait")) -> ()  [unwired: 1 out]
    "Gain (VoltsPerDegree/Second)" <- w325
    "Gain (VoltsPerDegree/Second) 2" <- w318
  }
  n148 = call "cRIO MAC.vi"() -> ("MAC Address"=→"MAC Address":string, "Personality"=w29:string)  [unwired: 2 in]
  "Personality" <- w29
  n149 = for {
    N: 1 -> [_]
    n150 = flat-sequence {
      frame #0 {
        n151 = Wait (ms)(milliseconds to wait=u32 1000) -> ()  [unwired: 1 out]
      }
      frame #1 {
        # "Initial condition is Robot Turret is aimed at Target.\nUse this to create the initial Target Bearing."
        n152 = global read "Robot Global Data.vi" "Turret Yaw"() -> (w340:dbl)
        n153 = global read "Robot Global Data.vi" "Robot Gyro"() -> (w339:dbl)
        n154 = Add(x=w340, y=w339) -> (x+y=w338:dbl)
        n155 = call "Gyro Angle.vi"("Mod"=360.0, "Input"=w338) -> ("Output"=w337:dbl)  [unwired: 9 in]
        n156 = global write "Robot Global Data.vi" "Target Bearing"(w337) -> ()
      }
    }
  }
  n157 = global write "Robot Global Data.vi" "Personality"(w29) -> ()
  n158 = call <vilib>:"WPI_RelayRefNum Registry Get.vi"("refnum name"="Compressor") -> ("RelayDevRef"=w68:T9)  [unwired: 9 in, 1 out]
  n159 = call <vilib>:"WPI_DigitalInputRefNum Registry Get.vi"("refnum name"="Compressor Switch") -> ("DigitalInputDevRef"=w76:T7)  [unwired: 9 in, 1 out]
  n160 = while {
    tunnel: w68 -> [w351]
    tunnel: w76 -> [w347]
    stop <- FALSE stop-if-true
    n161 = call <vilib>:"WPI_DriverStationGet Digital Input.vi"() -> ("Driver Station Digital Input (1-8)"=w345:bool[])  [unwired: 11 in]
    n162 = call <vilib>:"WPI_DigitalInputGetValue.vi"("DigitalInputDevRef"=w347) -> ("Value"=w346:bool)  [unwired: 8 in, 2 out]
    n163 = Index Array(array=w345, index=0) -> (element=w343:bool)
    n164 = Wait (ms)(milliseconds to wait=u32 300) -> ()  [unwired: 1 out]
    n165 = case shown="True" w343 {
      tunnel: [WPI_RelayValue."Off" ("RelayValue") w356] -> w349
      tunnel: [FALSE w355] -> w348
      tunnel: w346 -> [_ w355]
      frame False {
      }
      frame True {
        n166 = case shown="True" w355 {
          tunnel: [WPI_RelayValue."Forward" ("RelayValue") WPI_RelayValue."Off" ("RelayValue")] -> w356
          frame False {
          }
          frame True {
          }
        }
      }
    }
    n167 = call <vilib>:"WPI_RelaySet.vi"("RelayValue"=w349, "RelayDevRef"=w351) -> ()  [unwired: 8 in, 2 out]
    n168 = Not(x=w348) -> (.not. x?=w341:bool)
    "Compressor Running" <- w341
    n169 = Build Array(w341) -> (w342:bool[])
    n170 = call <vilib>:"WPI_DriverStationSet Digital Output.vi"("Driver Station Digital Output (1-8)"=w342) -> ()  [unwired: 10 in, 1 out]
  }
  n171 = disable-structure shown="Disabled" {
    frame Disabled {
      # "Measured Distance Between Break Beam Sensors installed on wood bracket"
      n172 = call <vilib>:"WPI_DigitalInputRefNum Registry Get.vi"("refnum name"="ball speed front") -> ("DigitalInputDevRef"=w363:T7)  [unwired: 9 in, 1 out]
      n173 = call <vilib>:"WPI_DigitalInputRefNum Registry Get.vi"("refnum name"="ball speed back") -> ("DigitalInputDevRef"=w362:T7)  [unwired: 9 in, 1 out]
      n174 = call "breakBeam.vi"("Falling Edge"=TRUE, "Rising Edge"=FALSE, "Distance between sensors(in)"=3.4375, "BreakBeam2"=w362, "BreakBeam1"=w363) -> ()  [unwired: 6 in, 1 out]
    }
    frame Enabled {
    }
  }
  n175 = call <vilib>:"WPI_CounterRefNum Registry Get.vi"("refnum name"="Shooter RPM") -> ("CounterDevRef"=w54:T27)  [unwired: 9 in, 1 out]
  n176 = disable-structure shown="Disabled" {
    disable-tunnel: [w369 _] -> w18
    disable-tunnel: [w368 _] -> w17
    frame Disabled {
      w368 = path "C:/tmp/Log Data12" ("datalog path (use dialog)")
      n177 = Open/Create/Replace File(file path (use dialog)=w368, operation (0:open)=T28."replace or create") -> ()  [unwired: 1 in, 6 out]
      n178 = Get Date/Time In Seconds() -> (seconds since 1Jan1904=w367:timestamp)
      n179 = To Double Precision Float(number=w367) -> (double precision float=w369:dbl)
    }
    frame Enabled {
    }
  }
  n180 = Get Date/Time In Seconds() -> (seconds since 1Jan1904=w36:timestamp)
  n181 = To Double Precision Float(number=w36) -> (double precision float=w35:dbl)
  n182 = call <vilib>:"WPI_MotorControlRefNum Registry Get.vi"("refnum name"="Shooter") -> ("MotorControlDevRef"=w96:T29)  [unwired: 9 in, 1 out]
  n183 = while {
    tunnel: w96 -> [w375]
    tunnel: w54 -> [w373]
    stop <- FALSE stop-if-true
    # "Run Sonar Loop for Fetch"
    n184 = global read "Robot Global Data.vi" "Enable Fetch"() -> (w372:bool)
    n185 = feedback #7() -> (w370:dbl)  [unwired: 1 in]
    n186 = case shown="True" w372 {
      tunnel: w375 -> [w386 w392]
      tunnel: w373 -> [w380 w390]
      tunnel: [w377 w391] -> w371
      tunnel: w370 -> [_ w391]
      frame False {
        n187 = global read "Robot Global Data.vi" "Shooter RPM Control"() -> (w385:dbl)
        n188 = call <vilib>:"WPI_CounterGet.vi"("CounterDevRef in"=w380) -> ("Period (sec)"=w378:dbl, "Stopped"=w379:bool)  [unwired: 5 in, 4 out]
        n189 = call "launcher.vi"("RPM Control"=w385, "Stall"=w379, "Period (sec)"=w378) -> ("RPM"=w384:dbl, "RPM Steady?"=w383:bool, "Motor Output"=w377:dbl)  [unwired: 2 in]
        "Motor Command" <- w377
        "RPM In Tol ?" <- w383
        n190 = global write "Robot Global Data.vi" "Shooter RPM Response"(w384) -> ()
        n191 = global write "Robot Global Data.vi" "Shooter Ready?"(w383) -> ()
        n192 = call "Stable.vi"("Pulse Width (sec)"="Shooter Stable Tol (sec)", "Signal Input"=w383) -> ("Stable"=w381:bool)  [unwired: 9 in]
        "RPM Stable ?" <- w381
        n193 = global write "Robot Global Data.vi" "Shooter Stable?"(w381) -> ()
        n194 = call "SimpleSetMotor.vi"("Output"=w377, "MotorControlDevRef"=w386) -> ()  [unwired: 8 in, 2 out]
      }
      frame True {
        # "If using Sonar control loop (during Fetch operation),\nturn off Shooter control loop for CPU load management\nand simply have Shooter motor 'coast' on last setting\ninstead of actively tracking a Distance-based command."
        n195 = call <vilib>:"WPI_CounterGet.vi"("CounterDevRef in"=w390) -> ("Period (sec)"=w387:dbl)  [unwired: 5 in, 5 out]
        n196 = Divide(x=60.0, y=w387) -> (x/y=w389:dbl)
        n197 = global write "Robot Global Data.vi" "Shooter RPM Response"(w389) -> ()
        n198 = call "SimpleSetMotor.vi"("Output"=w391, "MotorControlDevRef"=w392) -> ()  [unwired: 8 in, 2 out]
      }
    }
    n199 = feedback-in #7(w371) -> ()
    n200 = Wait (ms)(milliseconds to wait="Shooter Loop milliseconds") -> ()  [unwired: 1 out]
  }
  n201 = call <vilib>:"WPI_AnalogChannelRefNum Registry Get.vi"("refnum name"="Sonar Right") -> ("error out"=w23:errorcluster, "AIDeviceRef"=w22:T33)  [unwired: 1 in, 8 out]
  n202 = call <vilib>:"WPI_AnalogChannelRefNum Registry Get.vi"("refnum name"="Sonar Left") -> ("error out"=w19:errorcluster, "AIDeviceRef"=w20:T33)  [unwired: 1 in, 8 out]
  n203 = while {
    tunnel: w23 -> [w404]
    tunnel: w22 -> [w403]
    tunnel: w20 -> [w400]
    tunnel: w19 -> [w399]
    tunnel: w18 -> [w398]
    tunnel: w17 -> [w397]
    tunnel: w8 -> [w396]
    stop <- FALSE stop-if-true
    n204 = global read "Robot Global Data.vi" "Enable Fetch"() -> (w394:bool)
    n205 = Or(x=w394, y="Sonar Loop") -> (x .or. y?=w395:bool)
    n206 = case shown="True" w395 {
      tunnel: w404 -> [_ w470]
      tunnel: w403 -> [_ w469]
      tunnel: w400 -> [_ w468]
      tunnel: w399 -> [_ w467]
      tunnel: w398 -> [_ w462]
      tunnel: w397 -> [_ w461]
      tunnel: w396 -> [_ w406]
      frame False {
      }
      frame True {
        w449 = 3.75 ("Ball Radius")
        # "Capture State Machine"
        # "Prevent Fetch when have 3 balls"
        # "Sonar Seperation"
        # "Ball Radius"
        # "Lft Sonar"
        # "Rgt Sonar"
        # "Calc L & R distance to ball center"
        # "Calc error from centered"
        # "Perpindicular distance to object is (L*R)/Separation"
        # "Scaled for Readout in inches"
        n207 = disable-structure shown="Disabled" {
          disable-tunnel: w462 -> [w510 _]
          disable-tunnel: [w509 _] -> w432
          frame Disabled {
            # "Data Logging"
            n208 = Get Date/Time In Seconds() -> (seconds since 1Jan1904=w507:timestamp)
            n209 = To Double Precision Float(number=w507) -> (double precision float=w508:dbl)
            n210 = Subtract(x=w508, y=w510) -> (x-y=w509:dbl)
          }
          frame Enabled {
          }
        }
        n211 = flat-sequence {
          tunnel: [w480] -> w472
          tunnel: w470 -> [w479]
          tunnel: w469 -> [w478]
          tunnel: w468 -> [w477]
          tunnel: w467 -> [w476]
          tunnel: [w475] -> w466
          tunnel: [w473] -> w447
          frame #0 {
            n212 = Get Date/Time In Seconds() -> (seconds since 1Jan1904=w474:timestamp)
            n213 = call <vilib>:"WPI_AnalogChannelGetVoltage.vi"("error in (no error)"=w476, "AIDeviceRef"=w477) -> ("Voltage"=w475:dbl)  [unwired: 9 out]
            n214 = call <vilib>:"WPI_AnalogChannelGetVoltage.vi"("error in (no error)"=w479, "AIDeviceRef"=w478) -> ("Voltage"=w480:dbl)  [unwired: 9 out]
            n215 = To Double Precision Float(number=w474) -> (double precision float=w473:dbl)
          }
        }
        n216 = Multiply(x="Sonar Scale", y=w466) -> (x*y=w464:dbl)
        n217 = Multiply(x=w472, y="Sonar Scale") -> (x*y=w471:dbl)
        n218 = Add(x="Sonar Offset", y=w464) -> (x+y=w430:dbl)
        "Left Sonar" <- w430
        n219 = Add(x=w471, y="Sonar Offset") -> (x+y=w431:dbl)
        "Right Sonar" <- w431
        n220 = call "Rate Selective Filter.vi"("Hyster"="Hyster", "Rate Thresh"="Rate Thresh", "hi limit"=w406, "lo limit"=0.0, "Time"=w447, "Distance"=w430) -> ("Mode"=→"L Mode":bool, "OOR"=w443:bool, "Filtered"=w428:dbl)  [unwired: 1 in]
        "L Filtered" <- w428
        "L OOR" <- w443
        n221 = call "Rate Selective Filter.vi"("Hyster"="Hyster", "Rate Thresh"="Rate Thresh", "hi limit"=w406, "lo limit"=0.0, "Time"=w447, "Distance"=w431) -> ("Mode"=→"R Mode":bool, "OOR"=w444:bool, "Filtered"=w429:dbl)  [unwired: 1 in]
        "R Filtered" <- w429
        "R OOR" <- w444
        n222 = Bundle(w431, "Filtered"=w429) -> (→"R Sonar":cluster{dbl, "Filtered":dbl})  [unwired: 1 in]
        n223 = Bundle(w430, "Filtered"=w428) -> (→"L Sonar":cluster{dbl, "Filtered":dbl})  [unwired: 1 in]
        n224 = Not(x=w444) -> (.not. x?=w445:bool)
        n225 = Not(x=w443) -> (.not. x?=w446:bool)
        n226 = And(x=w445, y=w446) -> (x .and. y?=w441:bool)
        "Valid Target" <- w441
        n227 = Add(x=w449, y=w429) -> (x+y=w448:dbl)
        n228 = Add(x=w428, y=w449) -> (x+y=w450:dbl)
        n229 = Subtract(x=w450, y=w448) -> (x-y=w455:dbl)
        n230 = Multiply(x="Gain 2", y=w455) -> (x*y=w451:dbl)
        n231 = Multiply(x=w450, y=w448) -> (x*y=w453:dbl)
        n232 = Divide(x=w453, y=25.5 ("Sonar Separation")) -> (x/y=w410:dbl)
        n233 = expression code="-.0035*x*x+0.8091*x+2.594"(w410) -> (w409:dbl)
        "dist" <- w409
        n234 = Divide(x=w451, y="x") -> (x/y=w418:dbl)
        "error" <- w418
        n235 = Add(x="Balance 2", y=w418) -> (x+y=w420:dbl)
        n236 = Greater Than 0?(x=w418) -> (x > 0?=w421:bool)
        n237 = Select(t=w420, s=w421, f=w418) -> (s? t:f=w414:dbl)
        n238 = call "Stable.vi"("Pulse Width (sec)"="IR Delay (sec)", "Signal Input"=w441) -> ("Stable"=w408:bool)  [unwired: 9 in]
        "Stable" <- w408
        n239 = call "DSP.vi"("err"=w414, "Base"="Base") -> ("Right"=w412:dbl, "Left"=w413:dbl)  [unwired: 4 in]
        n240 = global read "Robot Global Data.vi" "INTAKE"() -> (w425:bool)
        "Intake" <- w425
        n241 = global read "Robot Global Data.vi" "Enable Fetch"() -> (w407:bool)
        n242 = call "Pulse Stretch & Delay.vi"("Delay (sec)"="Intake Delay (sec)", "In"=w425, "Width (sec)"=0.1) -> ("Out"=w422:bool)  [unwired: 2 in]
        n243 = Less Or Equal?(x=w409, y="Close") -> (x <= y?=w426:bool)
        "Close?" <- w426
        n244 = feedback #8(0) -> (w427:i32)
        n245 = disable-structure shown="Disabled" {
          disable-tunnel: w461 -> [w506 _]
          disable-tunnel: w432 -> [w505 _]
          disable-tunnel: w431 -> [w504 _]
          disable-tunnel: w430 -> [w503 _]
          disable-tunnel: w429 -> [w502 _]
          disable-tunnel: w428 -> [w501 _]
          disable-tunnel: w408 -> [w500 _]
          disable-tunnel: w427 -> [w499 _]
          disable-tunnel: w426 -> [w498 _]
          disable-tunnel: w425 -> [w497 _]
          disable-tunnel: w422 -> [w482 _]
          frame Disabled {
            n246 = global read "Robot Global Data.vi" "Enable Fetch"() -> (w486:bool)
            n247 = Boolean To (0,1)(Boolean=w486) -> (0, 1=w487:i16)
            n248 = To Double Precision Float(number=w487) -> (double precision float=w485:dbl)
            n249 = Boolean To (0,1)(Boolean=w482) -> (0, 1=w483:i16)
            n250 = To Double Precision Float(number=w483) -> (double precision float=w481:dbl)
            n251 = Boolean To (0,1)(Boolean=w498) -> (0, 1=w489:i16)
            n252 = Boolean To (0,1)(Boolean=w500) -> (0, 1=w490:i16)
            n253 = Boolean To (0,1)(Boolean=w497) -> (0, 1=w488:i16)
            n254 = To Double Precision Float(number=w489) -> (double precision float=w491:dbl)
            n255 = To Double Precision Float(number=w490) -> (double precision float=w493:dbl)
            n256 = To Double Precision Float(number=w499) -> (double precision float=w484:dbl)
            n257 = To Double Precision Float(number=w488) -> (double precision float=w492:dbl)
            n258 = Bundle "Bundle"(w505, w504, w503, "Filtered"=w502, "Filtered"=w501, w493, w491, w492, w481, w484, w485) -> (w494:T34)  [unwired: 1 out]
            n259 = Cluster To Array(cluster=w494) -> (array=w495:dbl[])
            n260 = call-poly <vilib>:"Write To Spreadsheet File.vi"("append to file? (new file:F)"=TRUE, "1D data"=w495, "file path (dialog if empty)"=w506) -> ()  [unwired: 3 in, 3 out]
          }
          frame Enabled {
          }
        }
        n261 = feedback #9() -> (w437:dbl)  [unwired: 1 in]
        n262 = case shown="1" w427 {
          tunnel: [w519 w531 w550 0 ("t")] -> w440
          tunnel: w408 -> [w515 w524 _ _]
          tunnel: w422 -> [_ _ w556 _]
          tunnel: w426 -> [_ w534 _ _]
          tunnel: [w514 w527 w546 w558] -> w435
          tunnel: [0.0 w529 w549 0.0] -> w438
          tunnel: w437 -> [_ _ w549 _]
          tunnel: [w513 w528 w546 w558] -> w434
          tunnel: w413 -> [_ w527 _ _]
          tunnel: w412 -> [_ w528 _ _]
          tunnel: "Base" -> [_ _ w546 _]
          tunnel: [FALSE TRUE FALSE FALSE] -> w433
          tunnel: w407 -> [w512 w523 w540 _]
          frame 0, Default {
            # "Wait for Target"
            n263 = global read "Robot Global Data.vi" "X Axis Drive Cmd"() -> (w514:dbl)
            n264 = global read "Robot Global Data.vi" "Y Axis Drive Cmd"() -> (w513:dbl)
            n265 = And(x=w512, y=w515) -> (x .and. y?=w516:bool)
            n266 = local write "Reset Sonar"(FALSE ("Reset Sonar")) -> ()
            n267 = Select(t=1, s=w516, f=0) -> (s? t:f=w519:i32)
          }
          frame 1 {
            # "Target Acquired, Steer using\nDifferential Sonar, unless lose target"
            n268 = And(x=w523, y=w524) -> (x .and. y?=w525:bool)
            n269 = Get Date/Time In Seconds() -> (seconds since 1Jan1904=w530:timestamp)
            n270 = To Double Precision Float(number=w530) -> (double precision float=w529:dbl)
            n271 = local write "Reset Sonar"(TRUE ("Reset Sonar")) -> ()
            n272 = Select(t=2, s=w534, f=1 ("t")) -> (s? t:f=w533:i32)
            n273 = Select(t=w533, s=w525, f=0) -> (s? t:f=w531:i32)
          }
          frame 2 {
            # "Target Close, Drive Straight,\nunless time out"
            n274 = Get Date/Time In Seconds() -> (seconds since 1Jan1904=w553:timestamp)
            n275 = To Double Precision Float(number=w553) -> (double precision float=w552:dbl)
            n276 = local write "Reset Sonar"(FALSE ("Reset Sonar")) -> ()
            n277 = Select(t=3, s=w556, f=2) -> (s? t:f=w548:i32)
            n278 = Not(x=w540) -> (.not. x?=w541:bool)
            n279 = Subtract(x=w552, y=w549) -> (x-y=w551:dbl)
            n280 = Greater?(x=w551, y="DS time") -> (0:w543:bool)
            n281 = Or(x=w541, y=w543) -> (x .or. y?=w542:bool)
            n282 = Select(t=0, s=w542, f=w548) -> (s? t:f=w550:i32)
            n283 = local write "Reset Sonar 4"(TRUE ("Reset Sonar")) -> ()
            n284 = local write "Reset Sonar 3"(TRUE ("Reset Sonar")) -> ()
          }
          frame 3 {
            w558 = 0.0
            # "Target Consumed, Stop,\ngo to Wait State"
          }
        }
        "Left Motor Sonar" <- w435
        "Right Motor Sonar" <- w434
        "Steering" <- w433
        "Sonar State" <- w440
        n285 = feedback-in #8(w440) -> ()
        n286 = feedback-in #9(w438) -> ()
        "hi limit" <- w406
      }
    }
    n287 = Wait Until Next ms Multiple(millisecond multiple=u32 10 ("milliseconds to wait")) -> ()  [unwired: 1 out]
  }
  n288 = call <vilib>:"WPI_RelayRefNum Registry Get.vi"("refnum name"="Sonar Kick") -> ("RelayDevRef"=w27:T9)  [unwired: 9 in, 1 out]
  n289 = while {
    shift-right: [w565] -> _
    shift-left: 0 -> [w564]
    tunnel: w27 -> [w566]
    stop <- TRUE continue-if-true
    n290 = global read "Robot Global Data.vi" "Kick Sonar"() -> (w561:bool)
    n291 = case shown="2" w564 {
      tunnel: w566 -> [w570 w572 w587 w591]
      tunnel: [1 2 w582 1] -> w565
      tunnel: "Dial" -> [_ w573 _ w588]
      tunnel: w561 -> [_ _ w581 _]
      frame 0, Default {
        # "Set pin to high impedance"
        # "Wait 250 ms to ensure sensor is up and running"
        n292 = call <vilib>:"WPI_RelaySet.vi"("RelayValue"=WPI_RelayValue."Off", "RelayDevRef"=w570) -> ()  [unwired: 8 in, 2 out]
        n293 = Wait (ms)(milliseconds to wait=u32 250) -> ()  [unwired: 1 out]
      }
      frame 1 {
        n294 = flat-sequence {
          tunnel: w572 -> [w576]
          tunnel: w573 -> [w577]
          tunnel: w572 -> [w578]
          frame #0 {
            # "Pull the pin high"
            n295 = call <vilib>:"WPI_RelaySet.vi"("RelayValue"=WPI_RelayValue."Forward", "RelayDevRef"=w576) -> ()  [unwired: 8 in, 2 out]
          }
          frame #1 {
            # "Keep the pin high for 30 us"
            n296 = call "Wait"("Count(uSec)"=w577) -> ()  [unwired: 1 out]
          }
          frame #2 {
            n297 = call <vilib>:"WPI_RelaySet.vi"("RelayValue"=WPI_RelayValue."Off", "RelayDevRef"=w578) -> ()  [unwired: 8 in, 2 out]
          }
        }
      }
      frame 2 {
        # "Reset State"
        # "Only reset on a rising edge"
        # "Set pin to high impedance"
        n298 = feedback-in #10(w581) -> ()
        n299 = feedback #10() -> (w580:bool)  [unwired: 1 in]
        n300 = call <vilib>:"WPI_RelaySet.vi"("RelayValue"=WPI_RelayValue."Off", "RelayDevRef"=w587) -> ()  [unwired: 8 in, 2 out]
        n301 = Greater?(x=w581, y=w580) -> (0:w585:bool)
        n302 = Select(t=3, s=w585, f=2) -> (s? t:f=w582:i32)
      }
      frame 3 {
        # "Pull pin low"
        n303 = call "Wait2"("Count(uSec)"=w588) -> ()  [unwired: 1 out]
        n304 = call <vilib>:"WPI_RelaySet.vi"("RelayValue"=WPI_RelayValue."Reverse", "RelayDevRef"=w591) -> ()  [unwired: 8 in, 2 out]
      }
    }
    n305 = Wait Until Next ms Multiple(millisecond multiple="ms multiple") -> ()  [unwired: 1 out]
    "Kick State" <- w564
  }
  n306 = Get Date/Time In Seconds() -> (seconds since 1Jan1904=w4:timestamp)
  n307 = To Double Precision Float(number=w4) -> (double precision float=w3:dbl)
  n308 = call-poly <vilib>:"Read From Spreadsheet File.vi"("delimiter (\\t)"="=" ("delimiter (\\t)"), "file path (dialog if empty)"=path "C:/tmp/Bridge Balance Settings.csv" ("datalog path (use dialog)")) -> ("all rows"=w5:string[][])  [unwired: 5 in, 4 out]
  n309 = call <vilib>:"WPI_DigitalInputRefNum Registry Get.vi"("refnum name"="Intake Break Beam") -> ("error out"=w92:errorcluster, "DigitalInputDevRef"=w91:T7)  [unwired: 9 in]
  n310 = for {
    tunnel: w5 -> [w596] mode=indexing
    n311 = Array To Cluster(array=w596) -> (cluster=w595:T35)
    n312 = Unbundle By Name(w595) -> ("all rows[0]"=w594:string, "all rows[1]"=w593:string)
    n313 = case shown="\"Shooter RPM OS\"" w594 {
      tunnel: w593 -> [_ w599 w601 w604 w607 w610 w613 w617]
      tunnel: 0.0 -> [_ w598 w600 w603 w606 w609 w612 w616]
      frame "", Default {
      }
      frame "K Prop" {
        n314 = Fract/Exp String To Number(string=w599, default (0 dbl)=w598) -> (number=→"K Prop 2":dbl)  [unwired: 2 in, 1 out]
      }
      frame "K Deriv" {
        n315 = Fract/Exp String To Number(string=w601, default (0 dbl)=w600) -> (number=→"K Deriv 2":dbl)  [unwired: 2 in, 1 out]
      }
      frame "Motor Add" {
        n316 = Fract/Exp String To Number(string=w604, default (0 dbl)=w603) -> (number=→"Motor Add":dbl)  [unwired: 2 in, 1 out]
      }
      frame "Coerce" {
        n317 = Fract/Exp String To Number(string=w607, default (0 dbl)=w606) -> (number=→"Coerce":dbl)  [unwired: 2 in, 1 out]
      }
      frame "Bal Tol" {
        n318 = Fract/Exp String To Number(string=w610, default (0 dbl)=w609) -> (number=→"Bal Tol":dbl)  [unwired: 2 in, 1 out]
      }
      frame "Tip Tol" {
        n319 = Fract/Exp String To Number(string=w613, default (0 dbl)=w612) -> (number=→"Tip Tol 2":dbl)  [unwired: 2 in, 1 out]
      }
      frame "Shooter RPM OS" {
        n320 = Fract/Exp String To Number(string=w617, default (0 dbl)=w616) -> (number=w615:dbl)  [unwired: 2 in, 1 out]
        n321 = global write "Robot Global Data.vi" "Shooter RPM Offset"(w615) -> ()
      }
    }
  }
  n322 = call <vilib>:"WPI_DigitalInputRefNum Registry Get.vi"("refnum name"="Break Beam A") -> ("error out"=w89:errorcluster, "DigitalInputDevRef"=w90:T7)  [unwired: 9 in]
  n323 = global write "Robot Global Data.vi" "Target Angle"(w57) -> ()
  n324 = global write "Robot Global Data.vi" "Valid Target ?"(w59) -> ()
  n325 = Bundle("Frame"=w58, "Distance"=w56, w57, "Valid Target"=w59) -> (w60:T36)  [unwired: 1 in]
  n326 = global write "Robot Global Data.vi" "Frame Num"(w58) -> ()
  n327 = global write "Robot Global Data.vi" "Target Distance"(w56) -> ()
  n328 = Type Cast(x=w60) -> (*(type *) &x=w62:string)  [unwired: 1 in]
  n329 = String Length(string=w62) -> (length=w61:i32)
  n330 = UDP Open(11:w67) -> (port=w65:refnum<k16>, 0:w66:errorcluster)  [unwired: 4 in, 1 out]
  n331 = disable-structure shown="Disabled" {
    disable-tunnel: [w618 _] -> w31
    frame Disabled {
      w618 = path "C:/tmp/Log Data8" ("datalog path (use dialog)")
      n332 = Open/Create/Replace File(file path (use dialog)=w618, operation (0:open)=T28."replace or create") -> ()  [unwired: 1 in, 6 out]
    }
    frame Enabled {
    }
  }
  n333 = while {
    tunnel: w66 -> [w627]
    tunnel: w65 -> [w626]
    tunnel: [w625] -> w64
    tunnel: [w624] -> w63
    tunnel: w61 -> [w622]
    tunnel: w60 -> [w621]
    stop <- FALSE stop-if-true
    n334 = UDP Read(connection ID=w626, max size (548)=548, timeout ms (25000)=-1, 8:w627) -> (data out=w623:string, error out=w624:errorcluster, 3:w625:refnum<k16>)  [unwired: 2 out]
    n335 = case shown="No Error" w624 {
      tunnel: w623 -> [w641 _]
      tunnel: w622 -> [w643 _]
      tunnel: w621 -> [w640 _]
      frame No Error {
        n336 = Type Cast(type=w640, x=w641) -> (*(type *) &x=w639:T36)
        n337 = String Length(string=w641) -> (length=w642:i32)
        n338 = Not Equal?(x=w642, y=w643) -> (x != y?=w638:bool)
        n339 = Unbundle(w639) -> ("Frame"=w637:i32, "Distance"=w636:dbl, w635:dbl, "Valid Target"=w632:bool)
        n340 = Not(x=w632) -> (.not. x?=w631:bool)
        n341 = Not A Number/Path/Refnum?(number/path/refnum=w636) -> (NaN/Path/Refnum?=w634:bool)
        n342 = Not A Number/Path/Refnum?(number/path/refnum=w635) -> (NaN/Path/Refnum?=w633:bool)
        n343 = Compound Arithmetic op=OR(w631, w634, w633, w638) -> (w630:bool)
        n344 = case shown="False" w630 {
          tunnel: w635 -> [w645 _]
          tunnel: w636 -> [w646 _]
          tunnel: w637 -> [w647 _]
          tunnel: w632 -> [w644 w648]
          frame False {
            n345 = global write "Robot Global Data.vi" "Frame Num"(w647) -> ()
            n346 = global write "Robot Global Data.vi" "Target Distance"(w646) -> ()
            n347 = global write "Robot Global Data.vi" "Target Angle"(w645) -> ()
            n348 = global write "Robot Global Data.vi" "Valid Target ?"(w644) -> ()
            "Frame" <- w647
            "Distance" <- w646
            "Angle 2" <- w645
            "Valid Target 2" <- w644
          }
          frame True {
            n349 = global write "Robot Global Data.vi" "Valid Target ?"(w648) -> ()
          }
        }
      }
      frame Error {
      }
    }
  }
  n350 = call <vilib>:"WPI_MotorControlRefNum Registry Get.vi"("refnum name"="Turret") -> ("MotorControlDevRef"=w71:T29)  [unwired: 9 in, 1 out]
  n351 = while {
    tunnel: w71 -> [w652]
    tunnel: w35 -> [w651]
    stop <- FALSE stop-if-true
    # "Run Sonar Loop for Fetch"
    n352 = global read "Robot Global Data.vi" "Enable Fetch"() -> (w649:bool)
    n353 = case shown="False" w649 {
      tunnel: w652 -> [w711 w736]
      tunnel: w651 -> [w693 _]
      frame False {
        # "Defeat Softstops"
        # "Soft Stops to prevent Turret from hitting Mechanical Hard Stops"
        n354 = global read "Robot Global Data.vi" "Op Button 7"() -> (w691:bool)
        n355 = global read "Robot Global Data.vi" "Turret Yaw Poition Command"() -> (w712:dbl)
        n356 = global read "Robot Global Data.vi" "Auto Target"() -> (w664:bool)
        n357 = global read "Robot Global Data.vi" "Valid Target ?"() -> (w688:bool)
        n358 = global read "Robot Global Data.vi" "Op Button 5"() -> (w696:bool)
        n359 = global read "Robot Global Data.vi" "Op Button 4"() -> (w695:bool)
        n360 = And(x=w688, y=w696) -> (x .and. y?=w690:bool)
        n361 = feedback #11() -> (w706:bool)  [unwired: 1 in]
        n362 = Select(t=w688, s=w664, f=FALSE) -> (s? t:f=w689:bool)
        n363 = Or(x=w691, y=w689) -> (x .or. y?=w692:bool)
        n364 = feedback-in #11(w692) -> ()
        n365 = Or(x=w690, y=w695) -> (x .or. y?=w694:bool)
        n366 = case shown="True" w694 {
          frame False {
          }
          frame True {
            # "Update Target Bearing on Request"
            n367 = disable-structure shown="Disabled" {
              frame Disabled {
                n368 = global read "Robot Global Data.vi" "Target Angle"() -> ()  [unwired: 1 out]
              }
              frame Enabled {
              }
            }
            n369 = global read "Robot Global Data.vi" "Robot Gyro"() -> (w715:dbl)
            n370 = global read "Robot Global Data.vi" "Turret Yaw"() -> (w716:dbl)
            n371 = Compound Arithmetic op=ADD(w716, 0.0 ("value"), w715) -> (w714:dbl)
            n372 = call "Gyro Angle.vi"("Mod"=360.0, "Input"=w714) -> ("Output"=w717:dbl)  [unwired: 9 in]
            n373 = global write "Robot Global Data.vi" "Target Bearing"(w717) -> ()
          }
        }
        n374 = global read "Robot Global Data.vi" "Turret Yaw Joystick Command"() -> (w657:dbl)
        n375 = Greater?(x=w692, y=w706) -> (0:w699:bool)
        n376 = call "turret.vi"("Ref Time"=w693, "reinitialize? (F)"=w699, "Auto Target ?"=w692, "Yaw Control"=w712) -> ("Motor Output"=w700:dbl, "Turret In Tol ?"=w709:bool)  [unwired: 5 in, 1 out]
        "Turret Ready?" <- w709
        n377 = Not(x="Test?") -> (.not. x?=w655:bool)
        n378 = global write "Robot Global Data.vi" "Turret Ready?"(w709) -> ()
        n379 = call "Stable.vi"("Pulse Width (sec)"="Turret Stable Tol (sec)", "Signal Input"=w709) -> ("Stable"=w654:bool)  [unwired: 9 in]
        "Turret Stable?" <- w654
        n380 = Select(t=w657, s=w655, f="Test Turret DB") -> (s? t:f=w659:dbl)
        n381 = Select(t=w700, s=w692, f=w659) -> (s? t:f=w670:dbl)
        "Motor Command" <- w670
        n382 = global write "Robot Global Data.vi" "Turret Stable?"(w654) -> ()
        n383 = global read "Robot Global Data.vi" "Turret Yaw"() -> (w661:dbl)
        n384 = local read "Read Right Limit"() -> (w705:dbl)
        n385 = local read "Read Left Limit"() -> (w704:dbl)
        n386 = Negate(x="Speed near Limit") -> (-x=w667:dbl)
        n387 = Less Or Equal?(x=w661, y=w704) -> (x <= y?=w697:bool)
        "Left Limit" <- w697
        n388 = Greater Or Equal?(x=w661, y=w705) -> (x >= y?=w698:bool)
        "Right Limit" <- w698
        n389 = Greater Than 0?(x=w670) -> (x > 0?=w676:bool)
        n390 = Subtract(x=w705, y="Near Limit (deg)") -> (x-y=w684:dbl)
        n391 = Less Than 0?(x=w670) -> (x < 0?=w681:bool)
        n392 = Add(x=w704, y="Near Limit (deg)") -> (x+y=w683:dbl)
        n393 = Greater Or Equal?(x=w661, y=w684) -> (x >= y?=w674:bool)
        n394 = Less Or Equal?(x=w661, y=w683) -> (x <= y?=w672:bool)
        n395 = In Range and Coerce(upper limit="Speed near Limit", x=w670, lower limit=0.0 ("upper limit")) -> (coerced(x)=w675:dbl)  [unwired: 1 out]
        n396 = And(x=w672, y=w676) -> (x .and. y?=w678:bool)
        n397 = And(x=w681, y=w674) -> (x .and. y?=w682:bool)
        n398 = In Range and Coerce(upper limit=0.0, x=w670, lower limit=w667) -> (coerced(x)=w680:dbl)  [unwired: 1 out]
        n399 = Select(t=w675, s=w678, f=w670) -> (s? t:f=w671:dbl)
        n400 = Select(t=w680, s=w682, f=w670) -> (s? t:f=w673:dbl)
        n401 = Select(t=w673, s=w674, f=w670) -> (s? t:f=w669:dbl)
        n402 = Select(t=w671, s=w672, f=w669) -> (s? t:f=w668:dbl)
        n403 = case shown="True" w697 {
          tunnel: [w719 w728] -> w685
          tunnel: w668 -> [w721 w729]
          tunnel: w698 -> [w720 w727]
          frame False {
            n404 = case shown="False" w720 {
              tunnel: w721 -> [w722 w724]
              tunnel: [w722 w723] -> w719
              frame False {
                # "At neither limit"
              }
              frame True {
                # "Only allow left travel"
                # "At RGT/ CW limit"
                n405 = Less Than 0?(x=w724) -> (x < 0?=w726:bool)
                n406 = Select(t=0.0, s=w726, f=w724) -> (s? t:f=w723:dbl)
              }
            }
          }
          frame True {
            # "At LFT / CCW limit"
            n407 = case shown="False" w727 {
              tunnel: w729 -> [w730 _]
              tunnel: [w731 0.0 ("Turret Yaw Control")] -> w728
              frame False {
                # "Only allow right travel"
                n408 = Greater Than 0?(x=w730) -> (x > 0?=w733:bool)
                n409 = Select(t=0.0, s=w733, f=w730) -> (s? t:f=w731:dbl)
              }
              frame True {
                # "Cannot Occur / be \nat both limits"
              }
            }
          }
        }
        n410 = global write "Robot Global Data.vi" "Left_Limit"(w697) -> ()
        n411 = global write "Robot Global Data.vi" "Right_Limit"(w698) -> ()
        n412 = Absolute Value(x=w670) -> (abs(x)=w707:dbl)
        n413 = global read "Robot Global Data.vi" "Op Button 11"() -> (w665:bool)
        n414 = Less Or Equal?(x=w707, y="Motor Cuttout") -> (x <= y?=w701:bool)
        "Motor is Cut Out" <- w701
        n415 = call "Latch Boolean.vi"("Boolean Input"=w665) -> ("Boolean Output"=w662:bool)
        "Softstop Override" <- w662
        n416 = Not(x=w662) -> (.not. x?=w663:bool)
        n417 = Select(t=w670, s=w662, f=w685) -> (s? t:f=w686:dbl)
        n418 = global write "Robot Global Data.vi" "Softstops Enabled"(w663) -> ()
        n419 = Select(t=0.0, s=w701, f=w686) -> (s? t:f=w660:dbl)
        "Motor Output" <- w660
        n420 = call "SimpleSetMotor.vi"("Output"=w660, "MotorControlDevRef"=w711) -> ()  [unwired: 8 in, 2 out]
      }
      frame True {
        # "If using Sonar control loop (during Fetch operation),\nturn off Turret control loop for CPU load management\nand simply have Turret motor off."
        n421 = call "SimpleSetMotor.vi"("Output"=0.0, "MotorControlDevRef"=w736) -> ()  [unwired: 8 in, 2 out]
      }
    }
    n422 = Wait Until Next ms Multiple(millisecond multiple=u32 30 ("milliseconds to wait")) -> ()  [unwired: 1 out]
  }
  n423 = call <vilib>:"WPI_DigitalInputRefNum Registry Get.vi"("refnum name"="Break Beam B") -> ("error out"=w83:errorcluster, "DigitalInputDevRef"=w84:T7)  [unwired: 9 in]
  n424 = disable-structure shown="Disabled" {
    disable-tunnel: [w737 _] -> w32
    frame Disabled {
      n425 = Get Date/Time In Seconds() -> (seconds since 1Jan1904=w738:timestamp)
      n426 = To Double Precision Float(number=w738) -> (double precision float=w737:dbl)
    }
    frame Enabled {
    }
  }
  n427 = disable-structure shown="Disabled" {
    frame Disabled {
      # "Driver Turn to Target"
      n428 = while {
        stop <- FALSE stop-if-true
        n429 = global read "Robot Global Data.vi" "Dr Button 4"() -> (w739:bool)
        "Turn" <- w739
        n430 = case shown="True" w739 {
          frame False {
          }
          frame True {
            n431 = global read "Robot Global Data.vi" "Robot Gyro"() -> (w748:dbl)
            "Robot Gyro" <- w748
            n432 = Bundle("Turn To"="Turn To", "Robot Gyro"=w748) -> (→"Bot Turn Control Response":cluster{"Turn To":dbl, "Robot Gyro":dbl})  [unwired: 1 out]
            n433 = Bundle("Prop"="Prop", "Int"="Int", "Deriv"="Deriv") -> (w749:cluster{"Prop":dbl, "Int":dbl, "Deriv":dbl})  [unwired: 1 out]
            n434 = Negate(x="Turn Rate") -> (-x=w747:dbl)
            n435 = Bundle("Turn Rate"="Turn Rate", w747) -> (w743:cluster{"Turn Rate":dbl, dbl})  [unwired: 1 out]
            n436 = call-poly <vilib>:"PID.vi"("output range"=w743, "PID gains"=w749, "process variable"=w748, "setpoint"="Turn To") -> ("output"=w742:dbl)  [unwired: 2 in, 5 out]
            "PID Output" <- w742
            "Output" <- w742
            n437 = global write "Robot Global Data.vi" "Driver Turn to Target"(w742) -> ()
          }
        }
        n438 = Wait (ms)(milliseconds to wait=u32 10) -> ()  [unwired: 1 out]
      }
    }
    frame Enabled {
    }
  }
  n439 = call <vilib>:"WPI_DigitalInputRefNum Registry Get.vi"("refnum name"="Prime Break Beam") -> ("error out"=w86:errorcluster, "DigitalInputDevRef"=w85:T7)  [unwired: 9 in]
  n440 = UDP Close(connection ID=w64, 8:w63) -> ()  [unwired: 2 out]
  n441 = call <vilib>:"WPI_MotorControlRefNum Registry Get.vi"("refnum name"="Intake") -> ("MotorControlDevRef"=w79:T29)  [unwired: 9 in, 1 out]
  n442 = call <vilib>:"WPI_RobotDriveRefNum Registry Get.vi"("refnum name"="RobotDrive") -> ("RobotDriveDevRef"=w33:T37)  [unwired: 1 in, 9 out]
  n443 = while {
    tunnel: w33 -> [w761]
    tunnel: w32 -> [w758]
    tunnel: w31 -> [w757]
    stop <- FALSE stop-if-true
    n444 = global read "Robot Global Data.vi" "Dr Button 4"() -> (w766:bool)
    "PB" <- w766
    n445 = global read "Robot Global Data.vi" "Personality"() -> (w755:string)
    n446 = Equal?(x=w755, y="Sting") -> (x = y?=w753:bool)
    n447 = feedback #12() -> (w762:dbl)  [unwired: 1 in]
    n448 = feedback #13() -> (w764:dbl)  [unwired: 1 in]
    n449 = feedback #14() -> (w759:bool)  [unwired: 1 in]
    n450 = case shown="False" w766 {
      tunnel: [w810 w862] -> w765
      tunnel: w764 -> [_ w862]
      tunnel: [w809 w861] -> w763
      tunnel: w762 -> [_ w861]
      tunnel: w761 -> [w808 w889]
      tunnel: [TRUE w874] -> w760
      tunnel: w759 -> [_ w873]
      tunnel: w758 -> [w805 _]
      tunnel: w757 -> [w804 _]
      tunnel: "error" -> [w789 _]
      tunnel: w753 -> [w774 _]
      frame False {
        w790 = 0.0 ("x")
        # "Drive, Fetch, and Balance"
        # "Remove some motor deadband"
        # "Auto-Balance"
        # "Tip Detect"
        # "Create Deadband"
        # "Keep track on Encoder values, last value before commanding 'Brake' will be the Control Loop Set Point"
        n451 = global read "Robot Global Data.vi" "Pitch Gyro"() -> (w782:dbl)
        n452 = Negate(x="Coerce") -> (-x=w779:dbl)
        n453 = global read "Robot Global Data.vi" "Right Wheel Encoder"() -> (w809:dbl)
        n454 = global read "Robot Global Data.vi" "Left Wheel Encoder"() -> (w810:dbl)
        n455 = Bundle("Coerce"="Coerce", w779) -> (w780:cluster{"Coerce":dbl, dbl})  [unwired: 1 out]
        n456 = Select(t="K Prop 2", s=w774, f=0.03) -> (s? t:f=w784:dbl)
        "K Prop" <- w784
        n457 = Select(t="Tip Tol 2", s=w774, f=1.9) -> (s? t:f=w786:dbl)
        "Tip Tol" <- w786
        n458 = Select(t="K Deriv 2", s=w774, f=0.001) -> (s? t:f=w772:dbl)
        "K Deriv" <- w772
        n459 = Bundle("f"=w784, "x"=0.0, "f"=w772) -> (w785:cluster{"f":dbl, "x":dbl, "f":dbl})  [unwired: 1 out]
        n460 = call-poly <vilib>:"PID.vi"("output range"=w780, "PID gains"=w785, "process variable"=w782, "setpoint"=0.0) -> ("output"=w773:dbl)  [unwired: 6 in, 1 out]
        n461 = Bundle("x"=w790, "Pitch Gyro"=w782) -> (→"Balance":cluster{"x":dbl, "Pitch Gyro":dbl})  [unwired: 1 out]
        n462 = call "TPD.vi"("Input"=w782, "Tol"=w786) -> (6:"Up ?"=w787:bool, 7:"Up ?"=w791:i64)  [unwired: 2 in, 4 out]
        "Up ?" <- w787
        n463 = Subtract(x=w790, y=w782) -> (x-y=w800:dbl)
        n464 = Absolute Value(x=w800) -> (abs(x)=w799:dbl)
        n465 = Less Or Equal?(x=w799, y="Bal Tol") -> (x <= y?=w802:bool)
        "In Tol?" <- w802
        n466 = Select(t=0.0, s=w802, f=w773) -> (s? t:f=w796:dbl)
        n467 = Absolute Value(x=w796) -> (abs(x)=w794:dbl)
        n468 = global read "Robot Global Data.vi" "Autonomous Drive"() -> (w788:bool)
        n469 = Add(x=w794, y="Motor Add") -> (x+y=w793:dbl)
        n470 = Multiply(x=w793, y=w791) -> (x*y=w795:dbl)
        n471 = disable-structure shown="Disabled" {
          disable-tunnel: w805 -> [w860 _]
          disable-tunnel: w804 -> [w859 _]
          disable-tunnel: w782 -> [w858 _]
          disable-tunnel: w795 -> [w857 _]
          disable-tunnel: w787 -> [w856 _]
          frame Disabled {
            # "Data Logging"
            n472 = Get Date/Time In Seconds() -> (seconds since 1Jan1904=w854:timestamp)
            n473 = To Double Precision Float(number=w854) -> (double precision float=w855:dbl)
            n474 = Boolean To (0,1)(Boolean=w856) -> (0, 1=w850:i16)
            n475 = Subtract(x=w855, y=w860) -> (x-y=w852:dbl)
            n476 = To Double Precision Float(number=w850) -> (double precision float=w848:dbl)
            n477 = Multiply(x=w848, y=10.0) -> (x*y=w847:dbl)
            n478 = Multiply(x=w857, y=10.0) -> (x*y=w844:dbl)
            n479 = Bundle "Bundle"(w852, "Pitch Gyro"=w858, w844, w847) -> (w849:cluster{dbl, "Pitch Gyro":dbl, dbl, dbl})  [unwired: 1 out]
            n480 = Cluster To Array(cluster=w849) -> (array=w851:dbl[])
            n481 = call-poly <vilib>:"Write To Spreadsheet File.vi"("append to file? (new file:F)"=TRUE, "1D data"=w851, "file path (dialog if empty)"=w859) -> ()  [unwired: 3 in, 3 out]
          }
          frame Enabled {
          }
        }
        n482 = global read "Robot Global Data.vi" "Enable Fetch"() -> (w807:bool)
        n483 = global read "Robot Global Data.vi" "Dr Button 3"() -> (w797:bool)
        n484 = case shown="False" w788 {
          tunnel: w808 -> [w815 w843]
          tunnel: w807 -> [w814 _]
          tunnel: w797 -> [w813 _]
          tunnel: w795 -> [w812 _]
          tunnel: w789 -> [w811 _]
          frame False {
            n485 = case shown="False" w814 {
              tunnel: w815 -> [w822 w832]
              tunnel: w812 -> [w818 _]
              tunnel: w813 -> [w819 _]
              tunnel: w811 -> [_ w831]
              frame False {
                # "Drive commands from Tele-Op"
                n486 = global read "Robot Global Data.vi" "X Axis Drive Cmd"() -> (w821:dbl)
                n487 = global read "Robot Global Data.vi" "Y Axis Drive Cmd"() -> (w820:dbl)
                n488 = case shown="True" w819 {
                  tunnel: [w824 0.0 ("X Axis Drive Cmd")] -> w817
                  tunnel: w821 -> [w824 _]
                  tunnel: [w823 w826] -> w816
                  tunnel: w820 -> [w823 _]
                  tunnel: w818 -> [_ w826]
                  frame False {
                    # "Normal Drive"
                  }
                  frame True {
                  }
                }
                "Drive" <- w816
                n489 = call-poly <vilib>:"WPI_RobotDriveArcadeDrive.vi"("Y axis value"=w816, "X axis value"=w817, "RobotDriveDevRef"=w822) -> ()  [unwired: 7 in, 2 out]
              }
              frame True {
                n490 = local read "Right Motor Sonar"() -> (w827:dbl)
                n491 = disable-structure shown="Disabled" {
                  disable-tunnel: w831 -> [w834 _]
                  frame Disabled {
                    w833 = 0.85 ("Base 2")
                    n492 = Add(x=w833, y=w834) -> ()  [unwired: 1 out]
                    n493 = Subtract(x=w833, y=w834) -> ()  [unwired: 1 out]
                  }
                  frame Enabled {
                  }
                }
                n494 = local read "Left Motor Sonar"() -> (w828:dbl)
                n495 = local read "Sonar State"() -> (w830:i32)
                n496 = Equal To 0?(x=w830) -> (x = 0?=w829:bool)
                n497 = case shown="False" w829 {
                  tunnel: w832 -> [w837 w840]
                  tunnel: w827 -> [w836 w838]
                  tunnel: w828 -> [w835 w839]
                  frame False {
                    n498 = call <vilib>:"WPI_RobotDriveTankDrive.vi"("Right axis value"=w836, "Left axis value"=w835, "RobotDriveDevRef"=w837) -> ()  [unwired: 7 in, 2 out]
                  }
                  frame True {
                    n499 = call-poly <vilib>:"WPI_RobotDriveArcadeDrive.vi"("Y axis value"=w838, "X axis value"=w839, "RobotDriveDevRef"=w840) -> ()  [unwired: 7 in, 2 out]
                  }
                }
              }
            }
          }
          frame True {
            # "These Globals are used to communicate Autonomous\ncommands from Tank Drive Mode.\nX Axis = Left Axis\nY Axis = Right Axis"
            n500 = global read "Robot Global Data.vi" "X Axis Drive Cmd"() -> (w842:dbl)
            n501 = global read "Robot Global Data.vi" "Y Axis Drive Cmd"() -> (w841:dbl)
            n502 = call <vilib>:"WPI_RobotDriveTankDrive.vi"("Right axis value"=w841, "Left axis value"=w842, "RobotDriveDevRef"=w843) -> ()  [unwired: 7 in, 2 out]
          }
        }
      }
      frame True {
        w902 = 1.0
        # "Encoder Parking Brake"
        # "Count Bumps"
        # "Create Joystick Dead Band"
        # "Send Motor Values for Braking"
        # "Sample Encoders"
        # "Control Drive motor dead band"
        n503 = global read "Robot Global Data.vi" "Y Axis Drive Cmd"() -> (w883:dbl)
        n504 = feedback-in #15(w873) -> ()
        n505 = feedback #15(FALSE) -> (w876:bool)
        n506 = Greater?(x=w873, y=w876) -> (0:w874:bool)
        n507 = In Range and Coerce(upper limit=0.5, x=w883, lower limit=-0.5) -> (In Range?=w886:bool)  [unwired: 1 out]
        n508 = global read "Robot Global Data.vi" "Left Wheel Encoder"() -> (w908:dbl)
        "Left Enc" <- w908
        n509 = global read "Robot Global Data.vi" "Right Wheel Encoder"() -> (w888:dbl)
        "Right Enc" <- w888
        n510 = Select(t=0.0 ("f"), s=w886, f=w883) -> (s? t:f=w868:dbl)
        n511 = Greater Than 0?(x=w868) -> (x > 0?=w880:bool)
        n512 = Less Than 0?(x=w868) -> (x < 0?=w881:bool)
        n513 = Bundle("Left Wheel Encoder"=w862, "Left Wheel Encoder"=w908) -> (→"Left Brake Control Response":T38)  [unwired: 1 out]
        n514 = call "Boolean Counter.vi"("Reset"=w874, "Initial Count"=i64 0, "Count Down"=w881, "Count Up"=w880) -> ("Count"=w878:i64)
        n515 = Multiply(x=w878, y="Brake Bump") -> (x*y=w879:i64)
        n516 = Add(x=w879, y=w861) -> (x+y=w866:dbl)
        n517 = Bundle("Prop 2"="Prop 2", "Int 2"="Int 2", "Deriv 2"="Deriv 2") -> (w904:T39)  [unwired: 1 out]
        n518 = call-poly <vilib>:"PID Output Rate Limiter.vi"("output rate (EGU/min)"="Bump rate", "initial output"=w861, "input (controller output)"=w866) -> ("output"=w867:dbl)  [unwired: 5 in, 1 out]
        "output 2" <- w867
        n519 = Negate(x=w902) -> (-x=w907:dbl)
        n520 = Add(x=w862, y=w879) -> (x+y=w865:dbl)
        n521 = Bundle(w902, w907) -> (w905:cluster{dbl, dbl})  [unwired: 1 out]
        n522 = call-poly <vilib>:"PID Output Rate Limiter.vi"("output rate (EGU/min)"="Bump rate", "initial output"=w862, "input (controller output)"=w865) -> ("output"=w864:dbl)  [unwired: 5 in, 1 out]
        "output" <- w864
        n523 = call-poly <vilib>:"PID.vi"("output range"=w905, "PID gains"=w904, "process variable"=w908, "setpoint"=w864) -> ("output"=w872:dbl)  [unwired: 2 in, 5 out]
        n524 = call-poly <vilib>:"PID.vi"("output range"=w905, "PID gains"=w904, "process variable"=w888, "setpoint"=w867) -> ("output"=w871:dbl)  [unwired: 2 in, 5 out]
        n525 = Negate(x="Brake Motor Deadband") -> (-x=w896:dbl)
        n526 = In Range and Coerce(upper limit="Brake Motor Deadband", x=w872, lower limit=w896) -> (In Range?=w870:bool)  [unwired: 1 out]
        n527 = In Range and Coerce(upper limit="Brake Motor Deadband", x=w871, lower limit=w896) -> (In Range?=w869:bool)  [unwired: 1 out]
        n528 = Sign(1:w872) -> (0:w903:dbl)
        n529 = Sign(1:w871) -> (0:w895:dbl)
        n530 = Multiply(x="Brake Motor Add", y=w895) -> (x*y=w894:dbl)
        n531 = Multiply(x=w903, y="Brake Motor Add") -> (x*y=w900:dbl)
        n532 = Add(x=w872, y=w900) -> (x+y=w899:dbl)
        n533 = Add(x=w894, y=w871) -> (x+y=w898:dbl)
        n534 = Select(t=0.0, s=w870, f=w899) -> (s? t:f=w891:dbl)
        "Left PID Out" <- w891
        "Left Output" <- w891
        n535 = Select(t=0.0, s=w869, f=w898) -> (s? t:f=w890:dbl)
        "Right Output" <- w890
        n536 = call <vilib>:"WPI_RobotDriveTankDrive.vi"("Right axis value"=w890, "Left axis value"=w891, "RobotDriveDevRef"=w889) -> ()  [unwired: 7 in, 2 out]
        "Left Wheel Encoder" <- w862
        "Right Wheel Encoder" <- w861
      }
    }
    n537 = feedback-in #12(w763) -> ()
    n538 = feedback-in #13(w765) -> ()
    n539 = feedback-in #14(w760) -> ()
    n540 = Wait (ms)(milliseconds to wait=u32 10) -> ()  [unwired: 1 out]
  }
  n541 = call <vilib>:"WPI_MotorControlRefNum Registry Get.vi"("refnum name"="Fire Conveyor") -> ("MotorControlDevRef"=w81:T29)  [unwired: 9 in, 1 out]
  n542 = call <vilib>:"WPI_MotorControlRefNum Registry Get.vi"("refnum name"="Lower Conveyor") -> ("MotorControlDevRef"=w73:T29)  [unwired: 9 in, 1 out]
  n543 = call <vilib>:"WPI_MotorControlRefNum Registry Get.vi"("refnum name"="Middle Conveyor") -> ("MotorControlDevRef"=w72:T29)  [unwired: 9 in, 1 out]
  n544 = while {
    tunnel: w92 -> [w955]
    tunnel: w91 -> [w954]
    tunnel: w90 -> [w952]
    tunnel: w89 -> [w951]
    tunnel: w86 -> [w949]
    tunnel: w85 -> [w948]
    tunnel: w84 -> [w947]
    tunnel: w83 -> [w946]
    tunnel: w81 -> [w932]
    tunnel: w79 -> [w943]
    tunnel: w73 -> [w937]
    tunnel: w72 -> [w933]
    tunnel: w3 -> [w928]
    tunnel: path "C:/tmp/Log Data21" ("datalog path (use dialog)") -> [w927]
    shift-right: [w923] -> _
    shift-left: dbl[][] [] ("array") -> [w922]
    stop <- FALSE stop-if-true
    # "Clear"
    # "Reverse"
    # "Fire"
    n545 = call <vilib>:"WPI_DigitalInputGetValue.vi"("error in (no error)"=w951, "DigitalInputDevRef"=w952) -> ("Value"=w915:bool)  [unwired: 7 in, 2 out]
    n546 = call "Pulse Stretch & Delay.vi"("Delay (sec)"=0.0, "In"=w915, "Width (sec)"="BB A Delay") -> ("Out"=w912:bool)  [unwired: 2 in]
    n547 = Not(x=w915) -> (.not. x?=w914:bool)
    n548 = call <vilib>:"WPI_DigitalInputGetValue.vi"("error in (no error)"=w946, "DigitalInputDevRef"=w947) -> ("Value"=w945:bool)  [unwired: 7 in, 2 out]
    n549 = call <vilib>:"WPI_DigitalInputGetValue.vi"("error in (no error)"=w955, "DigitalInputDevRef"=w954) -> ("Value"=w953:bool)  [unwired: 7 in, 2 out]
    n550 = call <vilib>:"WPI_DigitalInputGetValue.vi"("error in (no error)"=w949, "DigitalInputDevRef"=w948) -> ("Value"=w950:bool)  [unwired: 7 in, 2 out]
    n551 = Not(x=w945) -> (.not. x?=w925:bool)
    n552 = global write "Robot Global Data.vi" "BB B"(w925) -> ()
    n553 = Or(x=w914, y=w912) -> (x .or. y?=w913:bool)
    n554 = global write "Robot Global Data.vi" "BB A/B"(w913) -> ()
    n555 = Not(x=w953) -> (.not. x?=w941:bool)
    n556 = global write "Robot Global Data.vi" "INTAKE"(w941) -> ()
    n557 = Not(x=w950) -> (.not. x?=w924:bool)
    n558 = global write "Robot Global Data.vi" "PRIME"(w924) -> ()
    n559 = global read "Robot Global Data.vi" "Collector State Machine"() -> (w939:bool)
    n560 = global read "Robot Global Data.vi" "Op Button 5"() -> (w931:bool)
    n561 = global read "Robot Global Data.vi" "Op Button 6"() -> (w942:bool)
    n562 = call "Pulse Stretch & Delay.vi"("Delay (sec)"=0.0, "In"=w931, "Width (sec)"=0.5) -> ("Out"=w926:bool)  [unwired: 2 in]
    n563 = global write "Robot Global Data.vi" "Report Fire"(w926) -> ()
    n564 = case shown="True" w939 {
      tunnel: TRUE ("Intake Motor") -> [_ w1079]
      tunnel: w926 -> [_ w1078]
      tunnel: w942 -> [w1028 w1077]
      tunnel: w924 -> [w1024 w1076]
      tunnel: w925 -> [_ w1075]
      tunnel: w913 -> [_ w1074]
      tunnel: w941 -> [_ w1073]
      tunnel: FALSE ("Op Button 10") -> [_ w1072]
      tunnel: [w1041 w1071] -> w935
      tunnel: [w1039 w1068] -> w921
      tunnel: [w1037 w1067] -> w920
      tunnel: [w1023 w1070] -> w919
      frame False {
        # "Changed this to 5 from 4"
        # "Mid Conv Back"
        # "Mid Conv Forward"
        # "Fire"
        # "Prime"
        # "Lo Conv Back"
        # "Lo Conv Forward"
        # "Intake On"
        n565 = global read "Robot Global Data.vi" "Op Button 8"() -> (w1042:bool)
        n566 = global read "Robot Global Data.vi" "Op Button 5"() -> (w1035:bool)
        n567 = global read "Robot Global Data.vi" "Op Button 1"() -> (w1038:bool)
        n568 = global read "Robot Global Data.vi" "Op Button 2"() -> (w1040:bool)
        n569 = global read "Robot Global Data.vi" "Op Button 5"() -> (w1025:bool)
        n570 = case shown="False" w1042 {
          tunnel: "Intake Speed" -> [w1061 _]
          tunnel: [w1060 0.0 ("Fire Conv Speed")] -> w1041
          tunnel: w1028 -> [w1062 _]
          frame False {
            n571 = case shown="False" w1062 {
              tunnel: w1061 -> [w1063 _]
              tunnel: [w1063 -1.0 ("Fire Conv Speed")] -> w1060
              frame False {
              }
              frame True {
              }
            }
          }
          frame True {
          }
        }
        n572 = Not(x=w1024) -> (.not. x?=w1036:bool)
        n573 = case shown="False" w1038 {
          tunnel: [w1051 1.0 ("Fire Conv Speed")] -> w1037
          tunnel: w1028 -> [w1050 _]
          frame False {
            n574 = case shown="True" w1050 {
              tunnel: [0.0 ("Fire Conv Speed") -1.0 ("Fire Conv Speed")] -> w1051
              frame False {
              }
              frame True {
              }
            }
          }
          frame True {
          }
        }
        n575 = case shown="False" w1040 {
          tunnel: [w1056 1.0 ("Fire Conv Speed")] -> w1039
          tunnel: w1028 -> [w1055 _]
          frame False {
            n576 = case shown="True" w1055 {
              tunnel: [0.0 ("Fire Conv Speed") -1.0 ("Fire Conv Speed")] -> w1056
              frame False {
              }
              frame True {
              }
            }
          }
          frame True {
          }
        }
        n577 = And(x=w1035, y=w1036) -> (x .and. y?=w1034:bool)
        n578 = And(x=w1024, y=w1025) -> (x .and. y?=w1026:bool)
        n579 = case shown="True" w1034 {
          tunnel: "Prime Conv Speed" -> [_ w1049]
          tunnel: [0.0 ("Fire Conv Speed") w1049] -> w1032
          frame False {
          }
          frame True {
          }
        }
        n580 = case shown="True" w1026 {
          tunnel: "Fire Conv Speed" -> [_ w1047]
          tunnel: [0.0 ("Fire Conv Speed") w1047] -> w1031
          frame False {
          }
          frame True {
          }
        }
        n581 = case shown="False" w1028 {
          tunnel: [0.0 ("Fire Conv Speed") -1.0 ("Fire Conv Speed")] -> w1029
          frame False {
          }
          frame True {
          }
        }
        n582 = Add(x=w1032, y=w1031) -> (x+y=w1030:dbl)
        n583 = Add(x=w1029, y=w1030) -> (x+y=w1023:dbl)
      }
      frame True {
        n584 = call "Ball Collector SM 5.1.vi"("FIRE"=w1078, "REVERSE"=w1077, "Intake Motor"=w1079, "OVERRIDE"=w1072, "BB1"=w1073, "BB2"=w1074, "BB3"=w1075, "BB4"=w1076, "new behavior"=TRUE ("s")) -> ("Ball Count"=w1069:dbl, "Intake motor"=w1071:dbl, "Motor A 2"=w1068:dbl, "Motor B 3"=w1067:dbl, "Motor C"=w1070:dbl)  [unwired: 14 in]
        n585 = global write "Robot Global Data.vi" "Ball Count"(w1069) -> ()
      }
    }
    n586 = disable-structure shown="Disabled" {
      disable-tunnel: w928 -> [w983 _]
      disable-tunnel: w927 -> [w982 _]
      disable-tunnel: w926 -> [w981 _]
      disable-tunnel: w925 -> [w980 _]
      disable-tunnel: w924 -> [w979 _]
      disable-tunnel: [w961 _] -> w923
      disable-tunnel: w922 -> [w960 _]
      disable-tunnel: w921 -> [w959 _]
      disable-tunnel: w920 -> [w958 _]
      disable-tunnel: w919 -> [w957 _]
      disable-tunnel: w913 -> [w956 _]
      frame Disabled {
        n587 = Get Date/Time In Seconds() -> (seconds since 1Jan1904=w974:timestamp)
        n588 = To Double Precision Float(number=w974) -> (double precision float=w973:dbl)
        n589 = Boolean To (0,1)(Boolean=w981) -> (0, 1=w975:i16)
        n590 = Boolean To (0,1)(Boolean=w956) -> (0, 1=w976:i16)
        n591 = Boolean To (0,1)(Boolean=w980) -> (0, 1=w978:i16)
        n592 = Boolean To (0,1)(Boolean=w979) -> (0, 1=w977:i16)
        n593 = Subtract(x=w973, y=w983) -> (x-y=w972:dbl)
        n594 = To Double Precision Float(number=w975) -> (double precision float=w971:dbl)
        n595 = To Double Precision Float(number=w976) -> (double precision float=w970:dbl)
        n596 = To Double Precision Float(number=w978) -> (double precision float=w969:dbl)
        n597 = To Double Precision Float(number=w977) -> (double precision float=w968:dbl)
        n598 = Insert Into Array(array=dbl[] [], new element #1=w972, new element #2=w971, new element #3=w970, new element #4=w969, new element #5=w968, new element #6=w959, new element #7=w958, new element #8=w957) -> (w966:dbl[])  [unwired: 1 in]
        n599 = Insert Into Array(array=w960, new element=w966) -> (w961:dbl[][])  [unwired: 2 in]
        n600 = feedback #16(FALSE ("Save Data")) -> (w963:bool)
        n601 = feedback-in #16("Save Data") -> ()
        n602 = Greater?(x="Save Data", y=w963) -> (0:w964:bool)
        n603 = case shown="True" w964 {
          tunnel: w982 -> [_ w987]
          tunnel: w961 -> [_ w984]
          frame False {
          }
          frame True {
            n604 = call-poly <vilib>:"Write To Spreadsheet File.vi"("format (%.3f)"="%.6f", "append to file? (new file:F)"=FALSE, "2D data"=w984, "file path (dialog if empty)"=w987) -> ()  [unwired: 2 in, 3 out]
          }
        }
      }
      frame Enabled {
      }
    }
    n605 = disable-structure shown="Disabled" {
      frame Disabled {
        n606 = feedback #17() -> (w990:i32)  [unwired: 1 in]
        n607 = feedback #18() -> (w988:dbl)  [unwired: 1 in]
        n608 = case shown="2" w990 {
          tunnel: [w992 0.5 ("Motor C") "Motor C" 0.0 ("Motor C")] -> _
          tunnel: [w996 w998 w1009 w1018] -> w991
          tunnel: [0.0 w1002 w1012 0.0] -> w989
          tunnel: w988 -> [_ _ w1012 _]
          tunnel: _ -> [w992 _ _ _]
          frame 0, Default {
            n609 = global read "Robot Global Data.vi" "Op Button 1"() -> (w993:bool)
            n610 = Select(t=1, s=w993, f=0) -> (s? t:f=w996:i32)
          }
          frame 1 {
            n611 = global read "Robot Global Data.vi" "Op Button 2"() -> (w999:bool)
            n612 = Get Date/Time In Seconds() -> (seconds since 1Jan1904=w1003:timestamp)
            n613 = To Double Precision Float(number=w1003) -> (double precision float=w1002:dbl)
            n614 = Select(t=2, s=w999, f=1) -> (s? t:f=w998:i32)
          }
          frame 2 {
            n615 = Get Date/Time In Seconds() -> (seconds since 1Jan1904=w1014:timestamp)
            n616 = Add(x="time", y=w1012) -> (x+y=w1011:dbl)
            n617 = To Double Precision Float(number=w1014) -> (double precision float=w1010:dbl)
            n618 = Greater Or Equal?(x=w1010, y=w1011) -> (x >= y?=w1007:bool)
            n619 = Select(t=3, s=w1007, f=2) -> (s? t:f=w1009:i32)
          }
          frame 3 {
            n620 = global read "Robot Global Data.vi" "Op Button 3"() -> (w1016:bool)
            n621 = Select(t=0, s=w1016, f=3) -> (s? t:f=w1018:i32)
          }
        }
        n622 = feedback-in #17(w991) -> ()
        n623 = feedback-in #18(w989) -> ()
      }
      frame Enabled {
      }
    }
    n624 = call "SimpleSetMotor.vi"("Output"=w935, "MotorControlDevRef"=w943) -> ()  [unwired: 8 in, 2 out]
    n625 = call "SimpleSetMotor.vi"("Output"=w919, "MotorControlDevRef"=w932) -> ()  [unwired: 8 in, 2 out]
    n626 = To Single Precision Float(number=w935) -> (single precision float=w936:sgl)
    n627 = case shown="1" w936 {
      tunnel: [FALSE ("INTAKE Direction") TRUE ("INTAKE Direction")] -> w934
      frame -1, Default {
      }
      frame 1 {
      }
    }
    n628 = call "SimpleSetMotor.vi"("Output"=w921, "MotorControlDevRef"=w937) -> ()  [unwired: 8 in, 2 out]
    n629 = global write "Robot Global Data.vi" "INTAKE Direction"(w934) -> ()
    n630 = call "SimpleSetMotor.vi"("Output"=w920, "MotorControlDevRef"=w933) -> ()  [unwired: 8 in, 2 out]
    n631 = Wait (ms)(milliseconds to wait="Coll Loop TIme") -> ()  [unwired: 1 out]
  }
